vi "Convert_ERDs.vi"(0 "New Header?":bool, 2 "ERD Name":string[](array[string]), 5 "All_ERD_Data_Bundled_Brass In":T1, 7 "Array":T14[](array[typedef]) {"ERD Number" format="%.0x"}, 11 "Error In":errorcluster) -> (4 "All_ERD_Data_Bundled_Brass":T1, 15 "Error Out":errorcluster)   [LabVIEW 2021]
doc: "This VI parses the data from ERDs in correct format, units, etc. It handles all hex to dec conversions, hex to enum, and hex to boolean conversions.\n\nIf Raw Data from ERD is blank string, then it will output values from shift register."
uses:
  Common/LabVIEW GEA2 Toolkit/GEA3/type defs/ERD Read Data Out.ctl
  type defs/All_Bundled_Data.ctl
  type defs/Version.ctl
  type defs/ERD_Always_Show.ctl
  type defs/Brass Matrix.ctl
  type defs/CSV_File_String_Arrays.ctl
  type defs/Redundant.ctl
  type defs/Algorithms.ctl
  type defs/ATC_Data.ctl
  type defs/Fault Table Array.ctl
  type defs/Fault_Table_Info.ctl
  Dryer Tool (Commercial 2)/JL Dryer Tool Support/type defs/ERD_RJ45.ctl
  Dryer Tool (Commercial 2)/JL Dryer Tool Support/type defs/ERD_Commercial_Laundry.ctl
  type defs/BootloaderVersion.ctl
panel:
  out "x/y":dbl
  out "Data":string
  # "Wet Load Size"
  # "Dry Load Size"
  # "OOB"
  # "Wet Load Size"
  # "Dry Load Size"
  # "OOB"
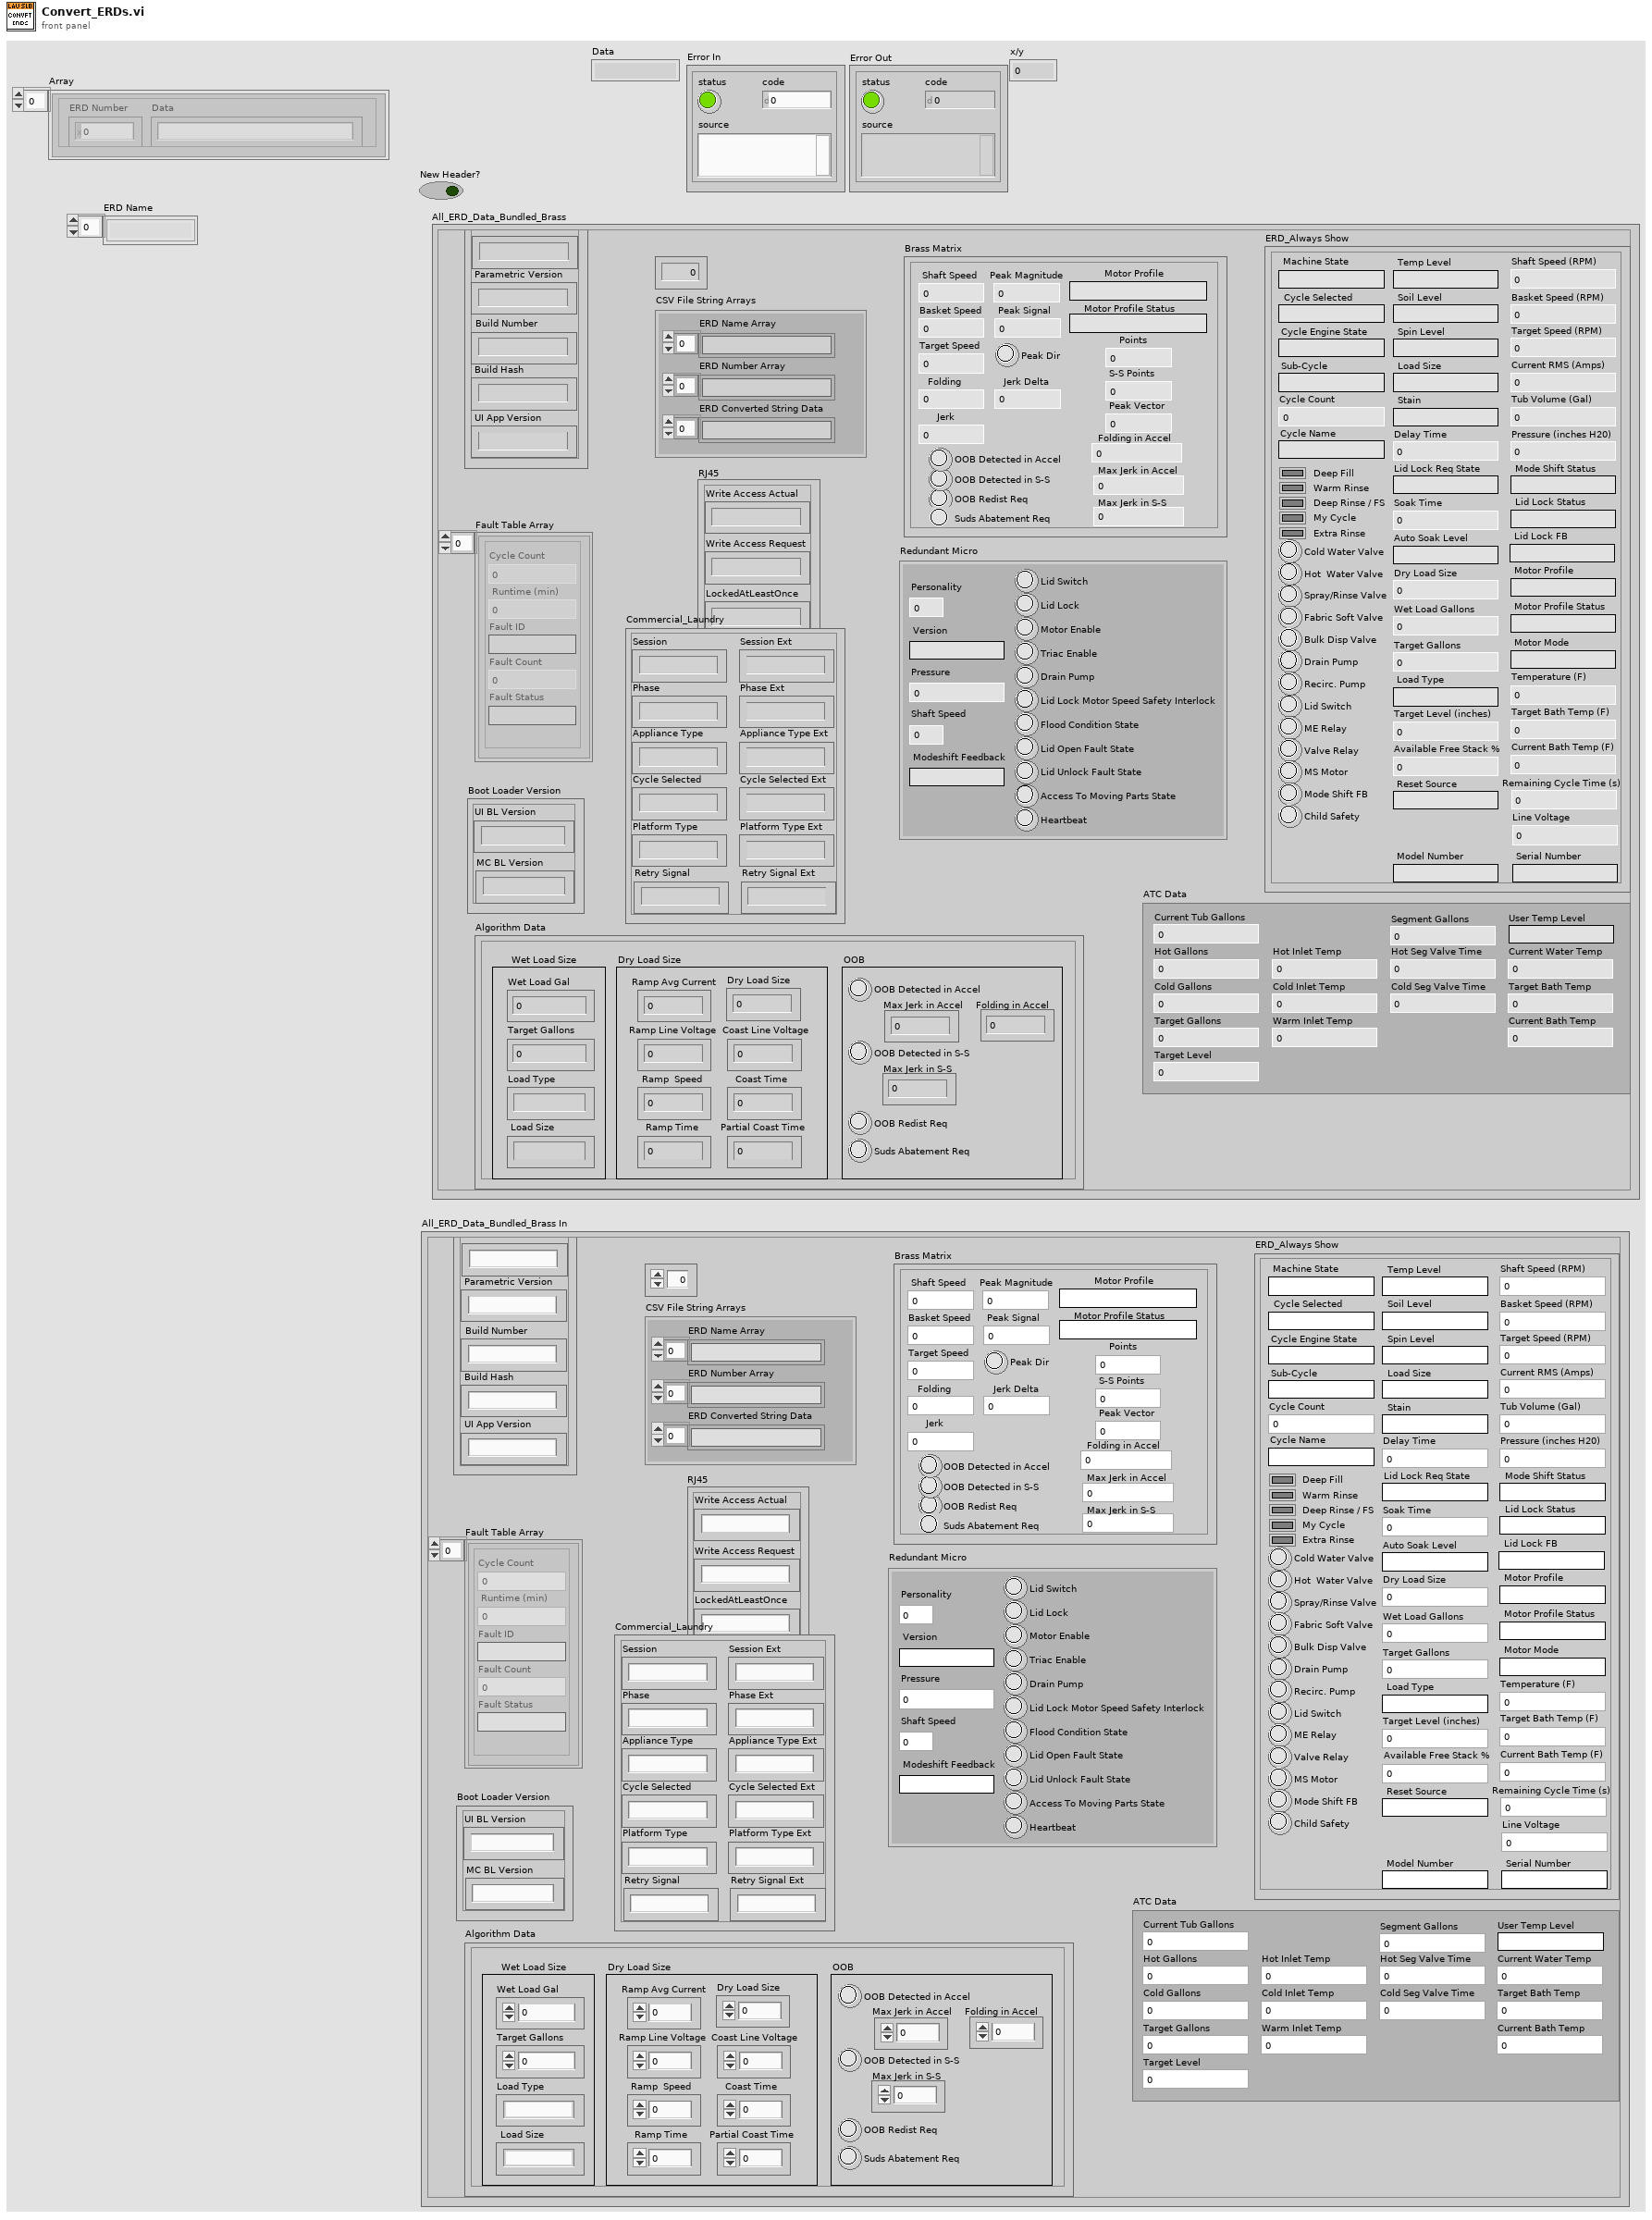
[diagram p1: front panel]
types:
  T1 = typedef "All_Bundled_Data.ctl" = cluster{"Software MC":T2, "ERD_Always Show":T3, "Personality Set":u8, "Brass Matrix":T4, "CSV File String Arrays":T5, "Redundant Micro":T6, "Algorithm Data":T7, "ATC Data":T8, "Fault Table Array ":T9, "RJ45":T11, "Commercial_Laundry":T12, "Boot Loader Version":T13}
  T2 = typedef "Version.ctl" = cluster{"Build Number":string, "Build Hash ":string, "Application Version":string, "Parametric Version":string, "UI App Version":string}
  T3 = typedef "ERD_Always_Show.ctl" = cluster{"Basket Speed (RPM)":u16, "Machine State":string, "Tub Volume (Gal)":dbl, "Pressure (inches H20)":dbl, "Lid Switch ":bool, "Current RMS (Amps)":dbl, "Cycle Selected":string, "Lid Lock Status":string, "Mode Shift Status":string, "Spray/Rinse Valve":bool, "Fabric Soft Valve":bool, "Drain Pump":bool, "Recirc. Pump":bool, "Cycle Engine State":string, "Hot  Water Valve":bool, "Cold Water Valve":bool, "Motor Profile":string, "Motor Profile Status":string, "Motor Mode":string, "ME Relay":bool, "Cycle Count":u32, "Deep Rinse / FS":bool, "My Cycle":bool, "Soil Level":string, "Spin Level":string, "Stain":string, "Temp Level":string, "Load Size":string, "Delay Time":u16, "Soak Time":u16, "Deep Fill":bool, "Warm Rinse":bool, "Auto Soak Level":string, "Extra Rinse":bool, "Wet Load Gallons":dbl, "Target Gallons":dbl, "Sub-Cycle":string, "Load Type":string, "Target Level (inches)":dbl, "Valve Relay":bool, "Dry Load Size":dbl, "Shaft Speed (RPM) ":u16, "MS Motor":bool, "Mode Shift FB":bool, "Target Bath Temp (F)":dbl, "Temperature (F)":dbl, "Current Bath Temp (F)":dbl, "Lid Lock FB":string, "Lid Lock Req State":string, "Remaining Cycle Time (s)":u32, "Available Free Stack %":u8, "Child Safety":bool, "Target Speed (RPM)":u16, "Reset Source":string, "Line Voltage":dbl, "Cycle Name":string, "Bulk Disp Valve":bool, "Model Number":string, "Serial Number":string}
  T4 = typedef "Brass Matrix.ctl" = cluster{"Shaft Speed":u16, "Folding":i32, "Jerk":i32, "Basket Speed":u16, "Target Speed":u16, "Peak Signal":u8, " Peak Magnitude":dbl, "Folding in Accel":i32, "Max Jerk in Accel":i32, "Max Jerk in S-S":i32, "Motor Profile Status":string, "Motor Profile":string, "OOB Redist Req":bool, "OOB Detected in S-S":bool, "OOB Detected in Accel":bool, "Suds Abatement Req ":bool, "Peak Dir":bool, "Peak Vector":dbl, "S-S Points":u8, "Points":u8, "Jerk Delta":i32}
  T5 = typedef "CSV_File_String_Arrays.ctl" = cluster{"ERD Number Array":string[], "ERD Name Array":string[], "ERD Converted String Data":string[]}
  T6 = typedef "Redundant.ctl" = cluster{"Version":string, "Personality":u8, "Pressure ":dbl, "Shaft Speed":u16, "Modeshift Feedback":string, "Lid Switch":bool, "Lid Lock":bool, "Triac Enable":bool, "Drain Pump":bool, "Lid Lock Motor Speed Safety Interlock":bool, "Flood Condition State":bool, "Lid Open Fault State":bool, "Access To Moving Parts State":bool, "Heartbeat":bool, "Motor Enable":bool, "Lid Unlock Fault State":bool}
  T7 = typedef "Algorithms.ctl" = cluster{"Wet Load Gal":dbl, "Target Gallons":dbl, "Load Type":string, "Load Size":string, "Coast Time":u16, "Ramp Time":u16, "Ramp  Speed":u16, "Ramp Avg Current":dbl, "OOB Redist Req":bool, "OOB Detected in S-S":bool, "Folding in Accel":i32, "Max Jerk in Accel":i32, "Max Jerk in S-S":i32, "OOB Detected in Accel":bool, "Partial Coast Time":u16, "Dry Load Size":dbl, "Ramp Line Voltage ":dbl, "Coast Line Voltage":dbl, "Suds Abatement Req ":bool}
  T8 = typedef "ATC_Data.ctl" = cluster{"Current Tub Gallons":dbl, "Hot Gallons":dbl, "Cold Gallons":dbl, "Target Gallons":dbl, "Current Water Temp":dbl, "Target Level":dbl, "Target Bath Temp":dbl, "Current Bath Temp ":dbl, "Cold Inlet Temp":dbl, "Hot Inlet Temp":dbl, "Warm Inlet Temp":dbl, "Hot Seg Valve Time":u16, "Cold Seg Valve Time ":u16, "User Temp Level":string, "Segment Gallons":dbl}
  T9 = typedef "Fault Table Array.ctl" = T10[]
  T10 = typedef "Fault_Table_Info.ctl" = cluster{"Cycle Count":u32, " Runtime (min) ":u32, "Fault Status":string, "Fault ID":string, "Fault Count":u16}
  T11 = typedef "ERD_RJ45.ctl" = cluster{"Write Access Actual":string, "Write Access Request":string, "LockedAtLeastOnce":string}
  T12 = typedef "ERD_Commercial_Laundry.ctl" = cluster{"Session":string, "Phase":string, "Appliance Type":string, "Cycle Selected":string, "Platform Type":string, "Retry Signal":string, "Session Ext":string, "Phase Ext":string, "Appliance Type Ext":string, "Cycle Selected Ext":string, "Platform Type Ext":string, "Retry Signal Ext":string}
  T13 = typedef "BootloaderVersion.ctl" = cluster{"UI BL Version":string, "MC BL Version":string}
  T14 = typedef "ERD Read Data Out.ctl" = cluster{"ERD Number":u16, "Data":string}
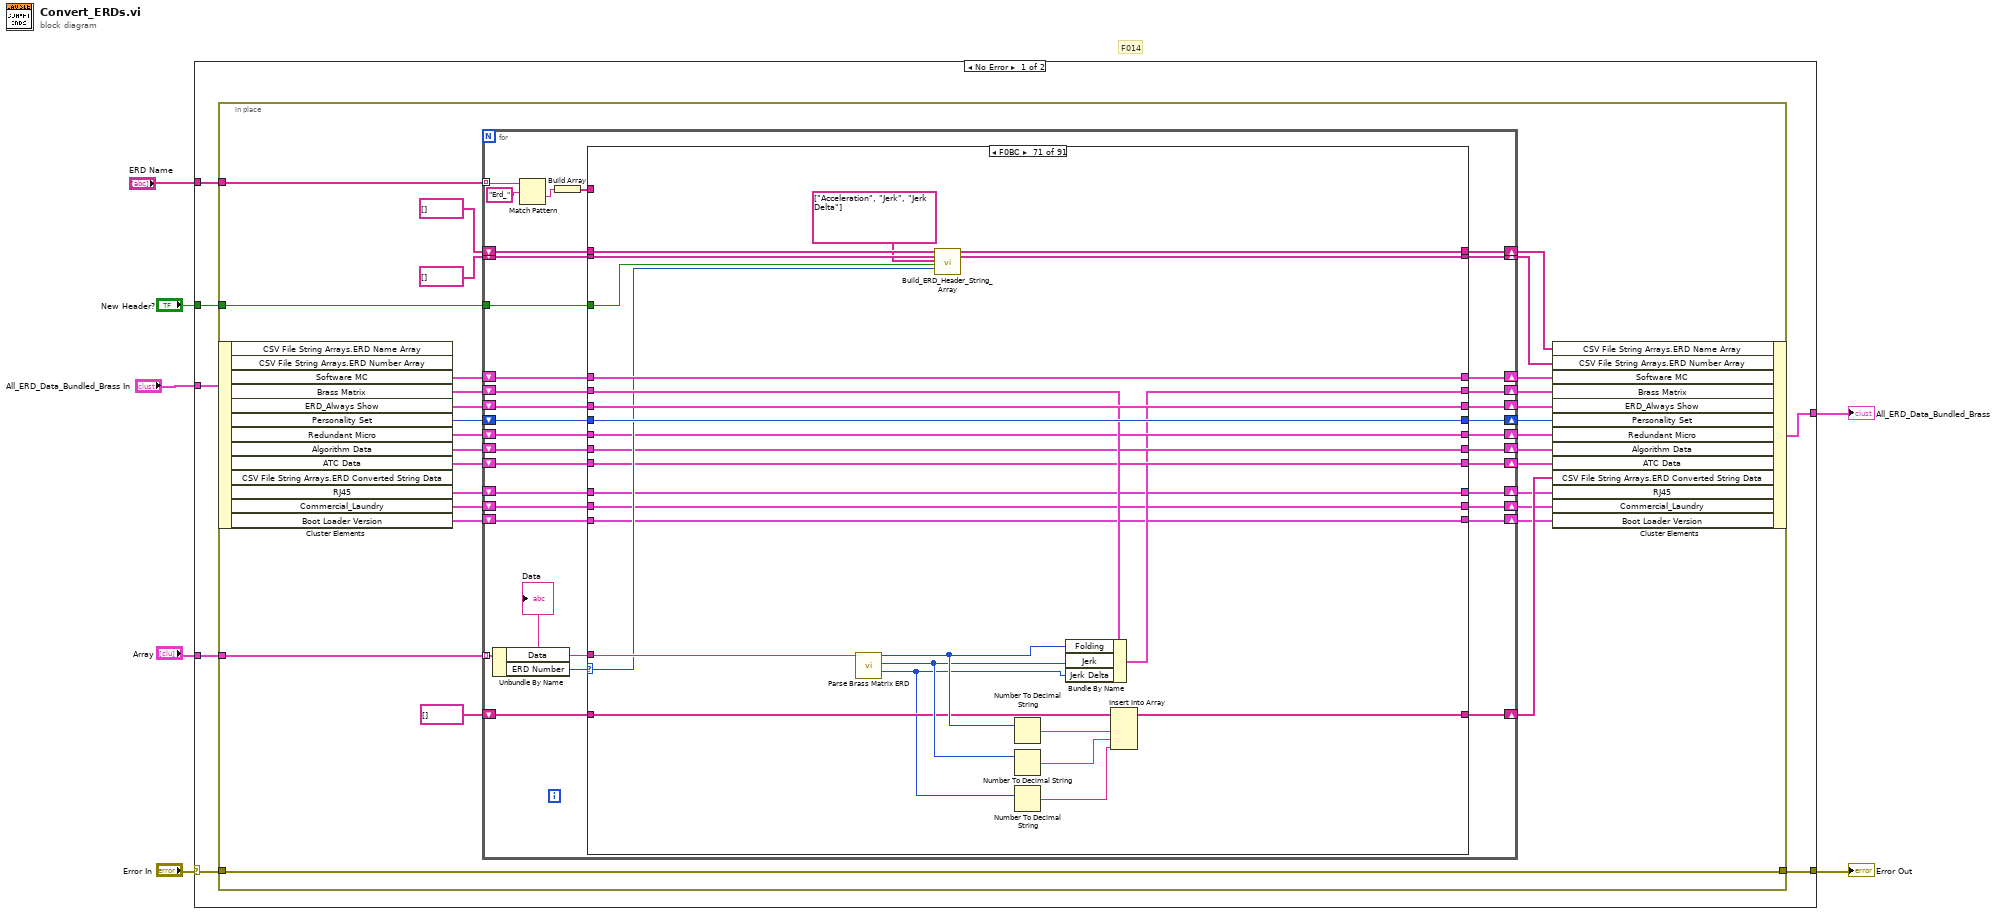
[diagram p0: block diagram]
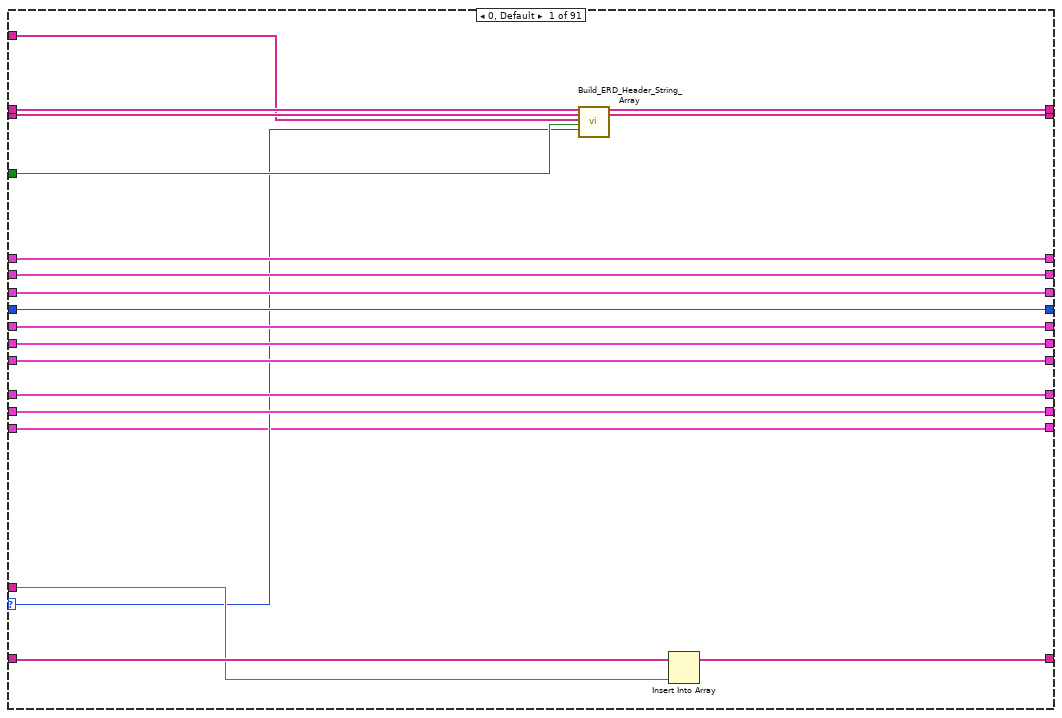
[diagram p2: hidden frame]
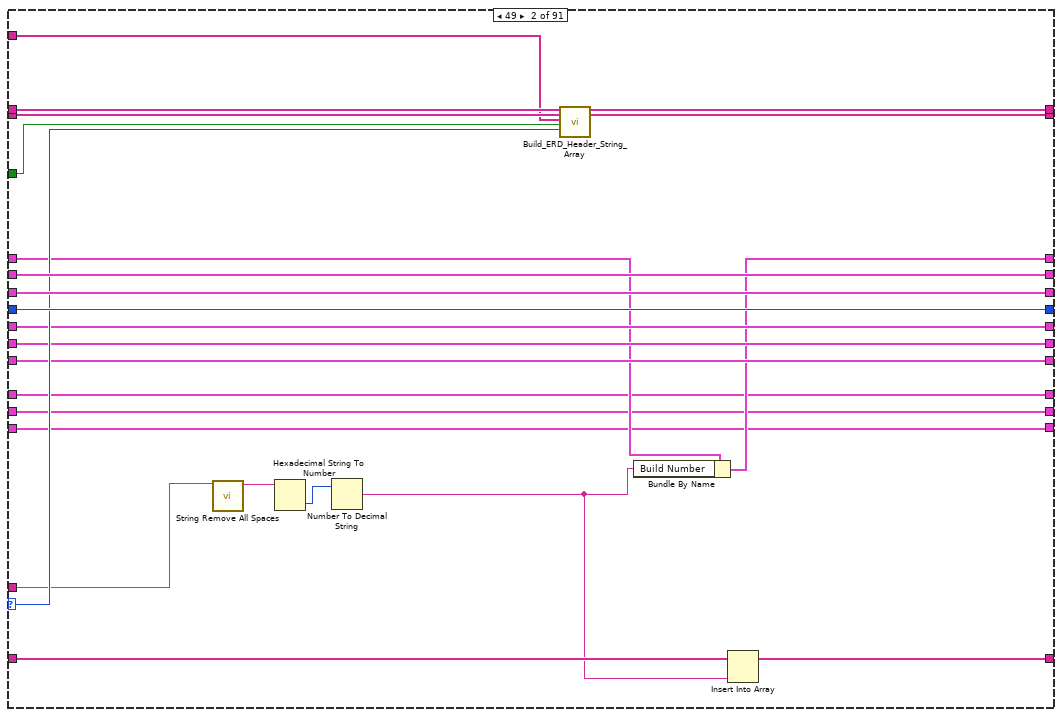
[diagram p3: hidden frame]
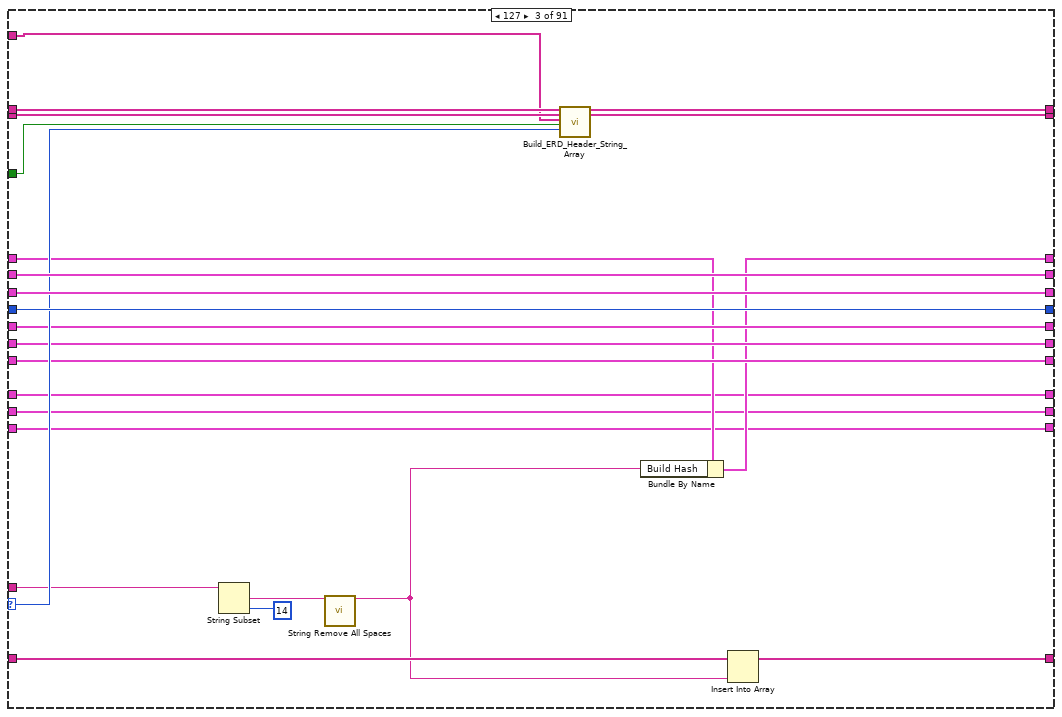
[diagram p4: hidden frame]
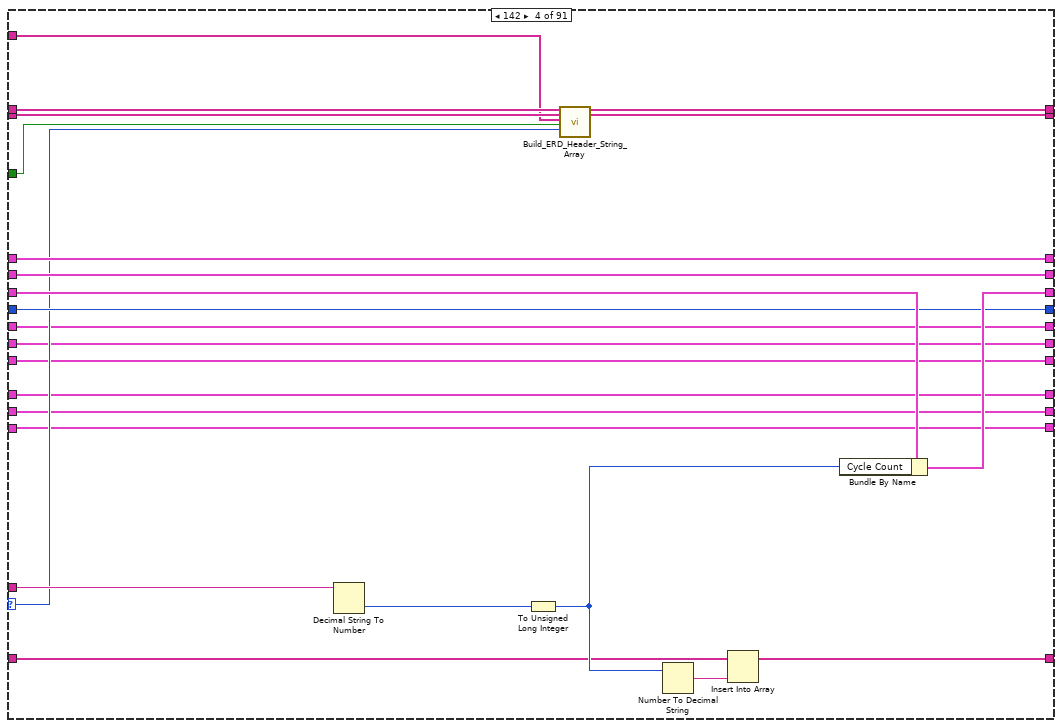
[diagram p5: hidden frame]
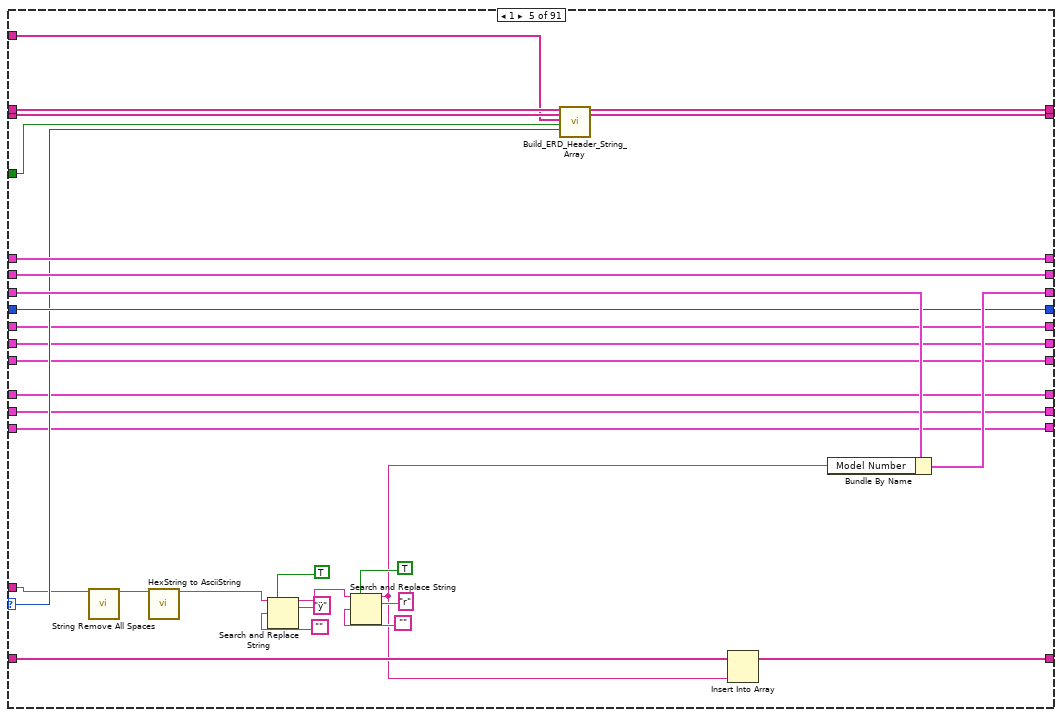
[diagram p6: hidden frame]
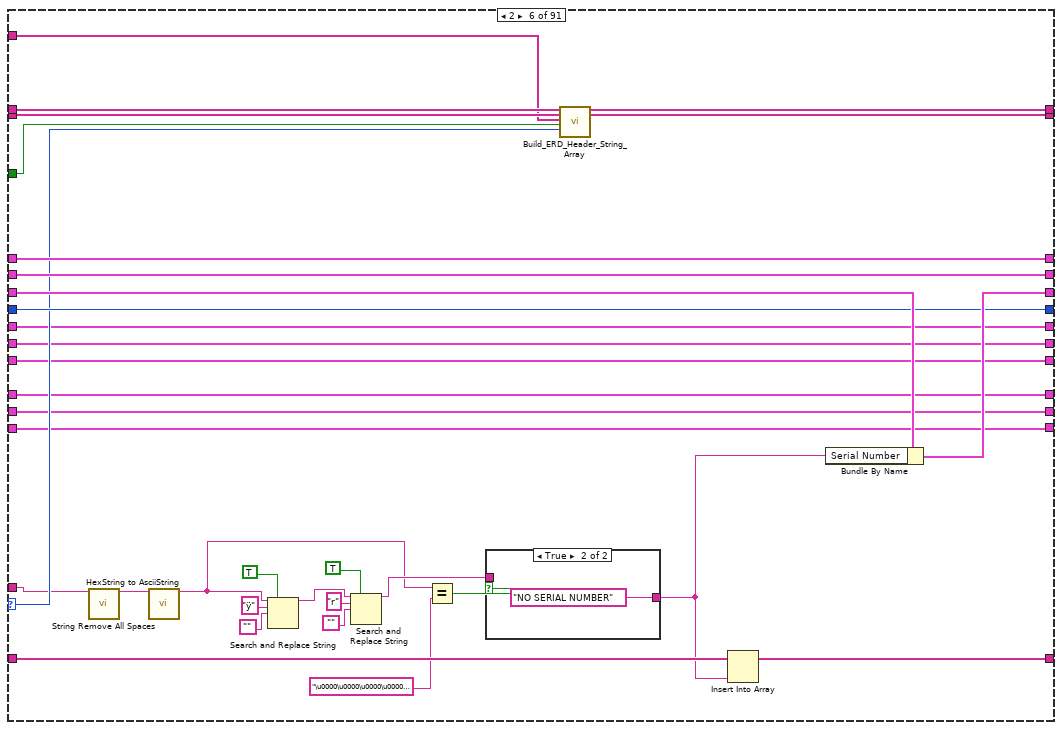
[diagram p7: hidden frame]
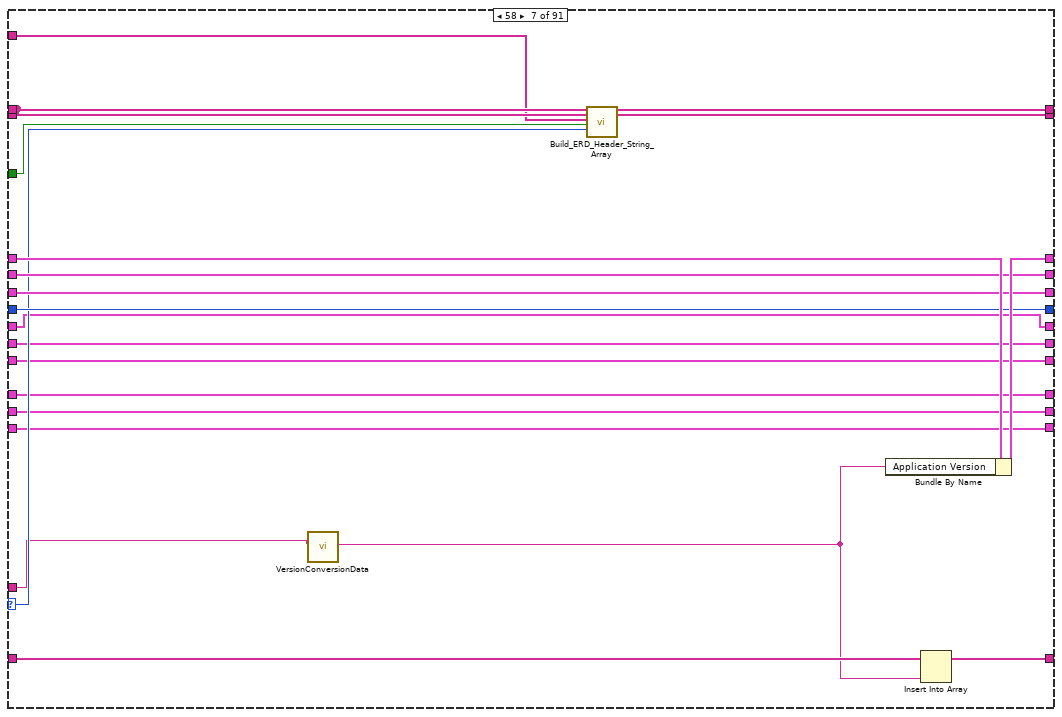
[diagram p9: hidden frame]
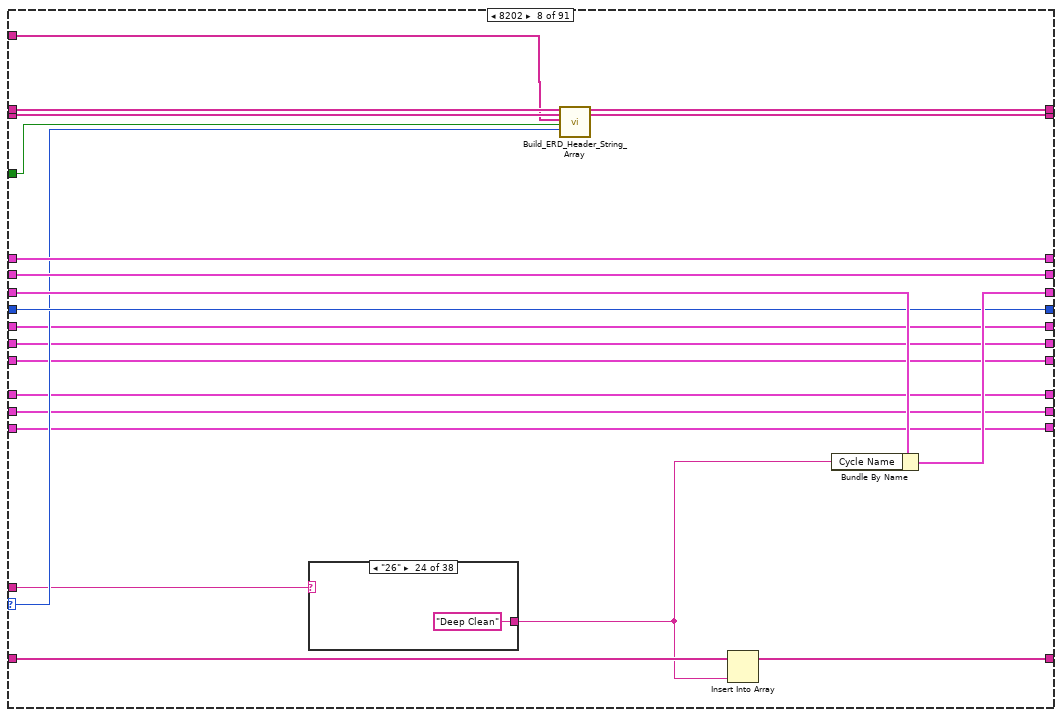
[diagram p10: hidden frame]
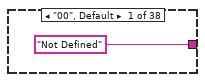
[diagram p11: hidden frame]
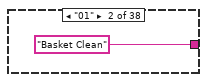
[diagram p12: hidden frame]
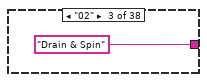
[diagram p13: hidden frame]
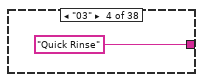
[diagram p14: hidden frame]
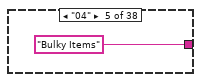
[diagram p15: hidden frame]
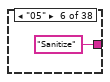
[diagram p16: hidden frame]
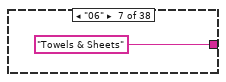
[diagram p17: hidden frame]
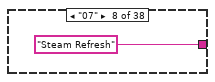
[diagram p18: hidden frame]
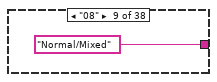
[diagram p19: hidden frame]
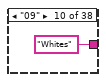
[diagram p20: hidden frame]
diagram:
  # "F014"
  n1 = case shown="No Error" "Error In" {
    selector: "Error In" -> [w11 w2792]
    tunnel: "Array" -> [w14 _]
    tunnel: [w12 w2791] -> w5
    tunnel: "All_ERD_Data_Bundled_Brass In" -> [w13 w2790]
    tunnel: [w10 w2790] -> w4
    tunnel: "New Header?" -> [w9 _]
    tunnel: "ERD Name" -> [w8 _]
    frame No Error {
      n2 = in-place {
        in-place-border: w14 -> [w44]
        in-place-border: [w40] -> w12
        in-place-border: w11 -> [w40]
        in-place-border: w9 -> [w33]
        in-place-border: w8 -> [w15]
        n3 = in-place-cluster #1(w13) -> ("Software MC"=w42:T2, "Brass Matrix"=w41:T4, "ERD_Always Show"=w43:T3, "Personality Set"=w36:u8, "Redundant Micro"=w26:T6, "Algorithm Data"=w25:T7, "ATC Data"=w23:T8, "RJ45"=w21:T11, "Commercial_Laundry"=w19:T12, "Boot Loader Version"=w17:T13)  [unwired: 3 out]
        n4 = for {
          tunnel: w44 -> [w78] mode=indexing
          shift-right: [w77] -> w37
          shift-left: w43 -> [w76]
          shift-right: [w74] -> w39
          shift-left: w42 -> [w75]
          shift-right: [w72] -> w38
          shift-left: w41 -> [w73]
          shift-right: [w69] -> w35
          shift-left: w36 -> [w70]
          shift-right: [w67] -> w28
          shift-left: string[] [] ("ERD String Data") -> [w68]
          tunnel: w33 -> [w66]
          shift-right: [w62] -> w29
          shift-left: string[] [] ("ERD String Data") -> [w65]
          shift-right: [w63] -> w30
          shift-left: string[] [] ("ERD String Data") -> [w64]
          shift-right: [w61] -> w27
          shift-left: w26 -> [w60]
          shift-right: [w58] -> w24
          shift-left: w25 -> [w59]
          shift-right: [w56] -> w22
          shift-left: w23 -> [w57]
          shift-right: [w54] -> w20
          shift-left: w21 -> [w55]
          shift-right: [w52] -> w18
          shift-left: w19 -> [w53]
          shift-right: [w50] -> w16
          shift-left: w17 -> [w51]
          tunnel: w15 -> [w47] mode=indexing
          n5 = Unbundle By Name(w78) -> ("Data"=w49:string, "ERD Number"=w71:u16)
          "Data" <- w49
          n6 = Match Pattern(string=w47, regular expression="Erd_") -> (after substring=w45:string)  [unwired: 1 in, 3 out]
          n7 = Build Array(w45) -> (w46:string[])
          n8 = case shown="F0BC" w71 {
            selector: w71 -> [w81 w114 w138 w159 w191 w225 w247 w270 w325 w349 w381 w401 w420 w444 w469 w494 w519 w550 w578 w610 w639 w672 w711 w733 w755 w783 w808 w841 w866 w900 w933 w955 w986 w1011 w1043 w1070 w1113 w1144 w1165 w1205 w1224 w1261 w1280 w1313 w1342 w1371 w1391 w1446 w1483 w1510 w1540 w1558 w1592 w1623 w1652 w1675 w1705 w1729 w1748 w1780 w1818 w1862 w1887 w1908 w1937 w1964 w2001 w2026 w2051 w2074 w2125 w2139 w2164 w2185 w2214 w2242 w2260 w2307 w2330 w2361 w2383 w2406 w2431 w2457 w2489 _ w2545 w2570 w2595 w2641 w2732]
            tunnel: w49 -> [w82 w102 w130 w170 w176 w206 w239 w264 w341 w362 w391 w392 w435 w458 w483 w508 w532 w560 w590 w622 w649 w685 w727 w741 w768 w800 w822 w827 w858 w892 w917 w969 w1004 w1030 w1058 w1084 w1104 w1156 w1182 w1192 w1242 w1246 w1300 w1304 w1333 w1382 w1411 w1459 w1495 w1502 w1552 w1575 w1604 w1614 w1644 w1691 w1715 w1739 w1767 w1790 w1828 w1847 w1875 w1922 w1950 w1980 w2015 w2040 w2065 w2088 w2128 w2152 w2179 w2204 w2229 w2252 w2277 w2286 w2344 w2368 w2379 w2402 w2440 w2453 w2502 w2512 w2536 w2561 w2586 w2609 w2700]
            tunnel: [w98 w122 w146 w168 w200 w234 w256 w279 w339 w363 w390 w411 w432 w459 w484 w509 w533 w561 w591 w621 w652 w687 w725 w748 w771 w798 w826 w854 w883 w913 w944 w967 w1003 w1025 w1056 w1095 w1131 w1154 w1181 w1217 w1240 w1273 w1298 w1332 w1361 w1387 w1433 w1475 w1494 w1528 w1550 w1576 w1607 w1641 w1670 w1694 w1718 w1743 w1765 w1807 w1845 w1873 w1897 w1925 w1947 w1982 w2013 w2038 w2063 w2097 w2131 w2153 w2177 w2202 w2227 w2255 w2282 w2319 w2342 w2373 w2398 w2421 w2444 w2467 w2504 w2513 w2554 w2579 w2604 w2650 w2741] -> w77
            tunnel: w76 -> [w98 w122 w146 w169 w201 w235 w256 w280 w340 w364 w390 w411 w434 w460 w485 w510 w534 w562 w592 w623 w651 w686 w726 w749 w772 w799 w821 w855 w884 w914 w945 w968 w1005 w1026 w1057 w1096 w1132 w1155 w1183 w1218 w1241 w1274 w1299 w1332 w1361 w1387 w1433 w1475 w1496 w1528 w1551 w1577 w1608 w1641 w1670 w1694 w1718 w1743 w1766 w1807 w1845 w1874 w1899 w1926 w1948 w1983 w2013 w2038 w2063 w2096 w2131 w2154 w2178 w2203 w2228 w2255 w2282 w2319 w2342 w2373 w2398 w2421 w2444 w2468 w2505 w2513 w2554 w2579 w2604 w2650 w2741]
            tunnel: w75 -> [w97 w108 w132 w167 w199 w233 w258 w278 w338 w361 w389 w413 w437 w457 w482 w507 w531 w559 w589 w620 w648 w684 w724 w747 w770 w797 w825 w853 w882 w912 w943 w966 w1002 w1027 w1055 w1082 w1130 w1153 w1180 w1216 w1239 w1272 w1297 w1331 w1360 w1386 w1432 w1474 w1498 w1527 w1549 w1574 w1603 w1640 w1669 w1693 w1717 w1742 w1764 w1808 w1846 w1872 w1898 w1920 w1949 w1979 w2014 w2039 w2064 w2087 w2130 w2151 w2176 w2201 w2226 w2254 w2281 w2318 w2343 w2372 w2397 w2420 w2443 w2482 w2501 w2516 w2541 w2566 w2591 w2638 w2729]
            tunnel: [w97 w107 w131 w167 w199 w233 w257 w278 w338 w361 w389 w412 w437 w457 w482 w507 w531 w559 w589 w620 w648 w684 w724 w747 w770 w797 w825 w853 w882 w912 w943 w966 w1002 w1027 w1055 w1082 w1130 w1153 w1180 w1216 w1239 w1272 w1297 w1331 w1360 w1386 w1432 w1474 w1498 w1527 w1549 w1574 w1603 w1640 w1669 w1693 w1717 w1742 w1764 w1808 w1846 w1872 w1898 w1920 w1949 w1979 w2014 w2039 w2064 w2087 w2130 w2151 w2176 w2201 w2226 w2254 w2281 w2318 w2343 w2372 w2397 w2420 w2443 w2482 w2501 w2516 w2541 w2566 w2591 w2638 w2729] -> w74
            tunnel: w73 -> [w96 w121 w145 w166 w198 w232 w255 w277 w337 w360 w388 w410 w436 w456 w481 w506 w530 w558 w588 w619 w647 w683 w723 w746 w769 w796 w824 w840 w881 w911 w942 w965 w1001 w1028 w1054 w1081 w1129 w1152 w1179 w1215 w1238 w1271 w1296 w1329 w1358 w1381 w1410 w1456 w1497 w1526 w1548 w1573 w1602 w1642 w1671 w1695 w1719 w1741 w1763 w1806 w1844 w1870 w1895 w1919 w1945 w1978 w2012 w2037 w2062 w2085 w2127 w2150 w2175 w2200 w2213 w2256 w2268 w2306 w2341 w2370 w2382 w2405 w2442 w2481 w2500 w2532 w2553 w2578 w2603 w2649 w2740]
            tunnel: [w96 w121 w145 w166 w198 w232 w255 w277 w337 w360 w388 w410 w436 w456 w481 w506 w530 w558 w588 w619 w647 w683 w723 w746 w769 w796 w824 w840 w881 w911 w942 w965 w1001 w1028 w1054 w1081 w1129 w1152 w1179 w1215 w1238 w1271 w1296 w1329 w1358 w1381 w1410 w1456 w1497 w1526 w1548 w1573 w1602 w1642 w1671 w1695 w1719 w1741 w1763 w1805 w1843 w1869 w1894 w1919 w1944 w1978 w2011 w2036 w2061 w2084 w2110 w2150 w2175 w2200 w2213 w2256 w2268 w2305 w2340 w2369 w2381 w2404 w2442 w2481 w2500 w2532 w2553 w2578 w2603 w2649 w2740] -> w72
            tunnel: w70 -> [w95 w120 w144 w165 w197 w231 w254 w276 w336 w359 w387 w409 w431 w455 w480 w505 w529 w557 w587 w618 w646 w682 w722 w745 w767 w795 w820 w852 w880 w910 w941 w964 w1000 w1024 w1053 w1080 w1128 w1151 w1178 w1214 w1237 w1270 w1295 w1328 w1357 w1380 w1409 w1455 w1493 w1525 w1547 w1572 w1599 w1638 w1667 w1690 w1714 w1738 w1762 w1789 w1827 w1871 w1896 w1918 w1946 w1977 w2010 w2035 w2060 w2086 w2129 w2149 w2174 w2199 w2225 w2251 w2276 w2317 w2339 w2371 w2395 w2418 _ w2480 w2499 w2531 w2552 w2577 w2602 w2648 w2739]
            tunnel: [w95 w120 w144 w165 w197 w231 w254 w276 w336 w359 w387 w409 w431 w455 w480 w505 w529 w557 w587 w618 w646 w682 w722 w745 w767 w795 w820 w852 w880 w910 w941 w964 w1000 w1024 w1053 w1080 w1128 w1151 w1178 w1214 w1237 w1270 w1295 w1328 w1357 w1380 w1409 w1455 w1493 w1525 w1547 w1572 w1599 w1638 w1667 w1690 w1714 w1738 w1762 w1789 w1827 w1871 w1896 w1918 w1946 w1977 w2010 w2035 w2060 w2086 w2129 w2149 w2174 w2199 w2225 w2251 w2276 w2317 w2339 w2371 w2395 w2418 w2427 w2480 w2499 w2531 w2552 w2577 w2602 w2648 w2739] -> w69
            tunnel: w68 -> [w87 w118 w142 w163 w195 w229 _ w274 w329 w353 w385 w405 w427 w448 w473 w498 w523 w554 w584 w614 w643 w676 w715 w739 w759 w787 w812 w845 w870 w904 w937 w959 w990 w1018 w1047 w1074 w1117 w1148 w1169 w1209 w1228 w1265 w1288 w1323 w1346 w1375 w1401 w1450 w1487 w1520 w1544 w1566 w1596 w1627 w1656 w1679 w1709 w1733 w1752 w1784 w1822 w1866 w1891 w1912 w1941 w1968 w2005 w2030 w2055 w2078 w2126 w2143 w2168 w2189 w2218 w2246 w2271 w2312 w2334 w2365 w2387 w2410 w2435 w2461 w2493 w2526 w2547 w2572 w2597 w2643 w2734]
            tunnel: [w85 w116 w140 w161 w193 w227 w249 w272 w327 w351 w383 w403 w425 w446 w471 w496 w521 w552 w582 w612 w641 w674 w713 w737 w757 w785 w810 w843 w868 w902 w935 w957 w988 w1016 w1045 w1072 w1115 w1146 w1167 w1207 w1226 w1263 w1286 w1321 w1344 w1373 w1399 w1448 w1485 w1518 w1542 w1564 w1594 w1625 w1654 w1677 w1707 w1731 w1750 w1782 w1820 w1864 w1889 w1910 w1939 w1966 w2003 w2028 w2053 w2076 w2123 w2141 w2166 w2187 w2216 w2244 w2269 w2310 w2332 w2363 w2385 w2408 w2433 w2459 w2491 w2523 w2543 w2568 w2593 w2639 w2730] -> w67
            tunnel: w66 -> [w89 w115 w139 w160 w192 w226 w248 w271 w326 w350 w382 w402 w424 w445 w470 w495 w520 w551 w579 w611 w640 w673 w712 w734 w756 w784 w809 w842 w867 w901 w934 w956 w987 w1012 w1044 w1071 w1114 w1145 w1166 w1206 w1225 w1262 w1281 w1314 w1343 w1372 w1392 w1447 w1484 w1511 w1541 w1559 w1593 w1624 w1653 w1676 w1706 w1730 w1749 w1781 w1819 w1863 w1888 w1909 w1938 w1965 w2002 w2027 w2052 w2075 w2124 w2140 w2165 w2186 w2215 w2243 w2261 w2309 w2331 w2362 w2384 w2407 w2432 w2458 w2490 w2525 w2546 w2571 w2596 w2642 w2733]
            tunnel: w65 -> [w88 w119 w143 w164 w196 w230 w251 w275 w330 w354 w386 w406 w428 w449 w474 w499 w524 w555 w585 w615 w644 w677 w716 w740 w760 w788 w813 w846 w871 w905 w938 w961 w991 w1019 w1048 w1075 w1118 w1149 w1170 w1210 w1229 w1266 w1289 w1324 w1347 w1376 w1402 w1451 w1488 w1521 w1545 w1567 w1597 w1628 w1657 w1680 w1710 w1734 w1753 w1785 w1823 w1867 w1892 w1913 w1942 w1969 w2006 w2031 w2056 w2079 w2122 w2144 w2169 w2190 w2219 w2247 w2272 w2313 w2335 w2366 w2388 w2411 w2436 w2462 w2494 w2527 w2548 w2573 w2598 w2644 w2735]
            tunnel: w64 -> [w83 w113 w137 w155 w190 w224 w253 w269 w333 w357 w380 w408 w430 w452 w477 w502 w527 w549 w581 w609 w638 w680 w719 w743 w764 w792 w817 w849 w875 w898 w927 w951 w995 w1015 w1042 w1069 w1122 w1139 w1174 w1201 w1233 w1258 w1284 w1317 w1353 w1367 w1394 w1441 w1481 w1514 w1538 w1562 w1591 w1632 w1661 w1684 w1701 w1725 w1756 w1776 w1816 w1858 w1882 w1906 w1932 w1973 w1998 w2023 w2048 w2073 w2114 w2137 w2161 w2194 w2222 w2238 w2264 w2303 w2327 w2355 w2391 w2414 w2429 w2456 w2488 w2522 w2538 w2563 w2588 w2637 w2728]
            tunnel: [w84 w112 w136 w154 w189 w223 w252 w268 w332 w356 w379 w407 w423 w451 w476 w501 w526 w548 w580 w608 w637 w679 w718 w742 w763 w791 w816 w848 w874 w897 w926 w952 w994 w1014 w1041 w1068 w1121 w1138 w1173 w1200 w1232 w1257 w1283 w1316 w1352 w1366 w1393 w1440 w1480 w1513 w1537 w1561 w1590 w1631 w1660 w1683 w1700 w1724 w1755 w1775 w1815 w1857 w1881 w1905 w1930 w1972 w1997 w2022 w2047 w2071 w2113 w2136 w2160 w2193 w2221 w2237 w2263 w2302 w2326 w2354 w2390 w2413 w2428 w2455 w2487 w2521 w2537 w2562 w2587 w2636 w2727] -> w63
            tunnel: [w86 w117 w141 w162 w194 w228 w250 w273 w328 w352 w384 w404 w426 w447 w472 w497 w522 w553 w583 w613 w642 w675 w714 w738 w758 w786 w811 w844 w869 w903 w936 w958 w989 w1017 w1046 w1073 w1116 w1147 w1168 w1208 w1227 w1264 w1287 w1322 w1345 w1374 w1400 w1449 w1486 w1519 w1543 w1565 w1595 w1626 w1655 w1678 w1708 w1732 w1751 w1783 w1821 w1865 w1890 w1911 w1940 w1967 w2004 w2029 w2054 w2077 w2119 w2142 w2167 w2188 w2217 w2245 w2270 w2311 w2333 w2364 w2386 w2409 w2434 w2460 w2492 w2524 w2544 w2569 w2594 w2640 w2731] -> w62
            tunnel: [w94 w111 w135 w153 w188 w222 w246 w267 w335 w358 w378 w400 w429 w454 w479 w504 w528 w556 w586 w617 w645 w681 w721 w744 w766 w794 w819 w851 w879 w909 w940 w963 w999 w1023 w1052 w1079 w1127 w1142 w1177 w1213 w1236 w1269 w1294 w1327 w1356 w1379 w1408 w1454 w1492 w1524 w1535 w1571 w1586 w1637 w1666 w1689 w1713 w1737 w1761 w1788 w1826 w1861 w1885 w1917 w1935 w1976 w2009 w2034 w2059 w2083 w2117 w2148 w2173 w2198 w2224 w2250 w2275 w2316 w2338 w2358 w2394 w2417 w2439 w2466 w2498 w2530 w2551 w2576 w2601 w2647 w2738] -> w61
            tunnel: w60 -> [w94 w111 w135 w153 w188 w222 w246 w267 w335 w358 _ w400 w429 w454 w479 w504 w528 w556 w586 w617 w645 w681 w721 w744 w766 w794 w819 w851 w879 w909 w940 w963 w999 w1023 w1052 w1079 w1127 w1142 w1177 w1213 w1236 w1269 w1294 w1327 w1356 w1379 w1408 w1454 w1492 w1524 w1535 w1571 w1586 w1637 w1666 w1689 w1713 w1737 w1761 w1788 w1826 w1861 w1885 w1917 w1935 w1976 w2009 w2034 w2059 w2083 w2117 w2148 w2173 w2198 w2224 w2250 w2275 w2316 w2338 w2358 w2394 w2417 w2439 w2466 w2498 w2530 w2551 w2576 w2601 w2647 w2738]
            tunnel: w59 -> [w93 w110 w134 w152 w187 w221 w245 w266 w324 w348 w377 w399 w419 w443 w468 w493 w518 w546 w577 w606 w635 w671 w710 w736 w754 w782 w807 w839 w878 w908 w930 w954 w998 w1022 w1051 w1078 w1126 w1141 w1176 w1212 w1235 w1268 w1293 w1326 w1355 w1378 w1407 w1453 w1491 w1523 w1534 w1570 w1585 w1635 w1664 w1687 w1704 w1728 w1759 w1779 w1814 w1860 w1884 w1916 w1934 w1975 w1996 w2021 w2046 w2082 w2116 w2147 w2172 w2197 w2212 w2241 w2267 w2315 w2325 w2357 w2392 w2415 w2438 w2465 w2497 w2529 w2550 w2575 w2600 w2646 w2737]
            tunnel: [w93 w110 w134 w152 w187 w221 w245 w266 w324 w348 w377 w399 w419 w443 w468 w493 w518 w546 w577 w605 w635 w671 w710 w736 w754 w782 w807 w838 w878 w908 w929 w953 w998 w1022 w1051 w1078 w1126 w1141 w1176 w1212 w1235 w1268 w1293 w1326 w1355 w1378 w1407 w1453 w1491 w1523 w1534 w1570 w1585 w1634 w1663 w1686 w1703 w1727 w1758 w1778 w1813 w1860 w1884 w1916 w1934 w1975 w1995 w2020 w2045 w2082 w2116 w2147 w2172 w2197 w2212 w2240 w2266 w2315 w2324 w2357 w2392 w2415 w2438 w2465 w2497 w2529 w2550 w2575 w2600 w2646 w2737] -> w58
            tunnel: w57 -> [w92 w109 w133 w151 w186 w220 w244 w265 w323 w347 w376 w398 w418 w442 w467 w492 w517 w545 w576 w607 w634 w670 w709 w735 w753 w781 w806 w836 w877 w907 w932 w962 w997 w1021 w1050 w1077 w1125 w1140 w1175 w1204 w1234 w1260 w1292 w1320 w1351 w1370 w1405 w1444 w1490 w1517 w1533 w1569 w1584 w1636 w1665 w1688 w1712 w1736 w1760 w1787 w1825 w1859 w1883 w1915 w1933 w1974 w2008 w2033 w2058 w2081 w2115 w2146 w2171 w2196 w2210 w2249 w2274 w2314 w2337 w2356 w2393 w2416 w2437 w2464 w2496 w2528 w2549 w2574 w2599 w2645 w2736]
            tunnel: [w92 w109 w133 w151 w186 w220 w244 w265 w323 w347 w376 w398 w418 w442 w467 w492 w517 w545 w575 w607 w634 w670 w709 w735 w753 w781 w806 w836 w877 w907 w931 w962 w997 w1021 w1050 w1077 w1124 w1140 w1175 w1203 w1234 w1259 w1291 w1319 w1350 w1369 w1406 w1445 w1490 w1516 w1533 w1569 w1584 w1636 w1665 w1688 w1712 w1736 w1760 w1787 w1825 w1859 w1883 w1915 w1933 w1974 w2008 w2033 w2058 w2081 w2115 w2146 w2171 w2196 w2210 w2249 w2274 w2314 w2337 w2356 w2393 w2416 w2437 w2464 w2496 w2528 w2549 w2574 w2599 w2645 w2736] -> w56
            tunnel: w55 -> [w91 w106 w126 w150 w174 w211 w243 w262 w322 w346 w375 w397 w417 w441 w466 w491 w516 w544 w573 w603 w633 w669 w708 w732 w752 w780 w805 w835 w865 w895 w924 w949 w985 w1010 w1039 w1065 w1112 w1136 w1164 w1199 w1223 w1254 w1279 w1312 w1341 w1364 w1390 w1436 w1478 w1509 w1532 w1557 w1582 w1622 w1651 w1674 w1698 w1722 w1746 w1773 w1811 w1855 w1879 w1903 w1929 w1963 w1993 w2018 w2043 w2068 w2107 w2134 w2159 w2184 w2209 w2235 w2259 w2287 w2322 w2347 w2378 w2401 w2426 w2447 w2485 w2520 w2540 w2565 w2590 w2632 w2723]
            tunnel: [w91 w106 w126 w150 w174 w211 w243 w262 w322 w346 w375 w397 w417 w441 w466 w491 w516 w544 w573 w603 w633 w669 w708 w732 w752 w780 w805 w835 w865 w895 w924 w949 w985 w1010 w1039 w1065 w1112 w1136 w1164 w1199 w1223 w1254 w1279 w1312 w1341 w1364 w1390 w1436 w1478 w1509 w1532 w1557 w1582 w1622 w1651 w1674 w1698 w1722 w1746 w1773 w1811 w1855 w1879 w1903 w1929 w1963 w1993 w2018 w2043 w2068 w2107 w2134 w2159 w2184 w2209 w2235 w2259 w2287 w2322 w2347 w2378 w2401 w2426 w2447 w2485 w2520 w2539 w2564 w2589 w2632 w2723] -> w54
            tunnel: w53 -> [w90 w105 w125 w149 w173 w210 w242 w261 w321 w345 w374 w396 w416 w440 w465 w490 w515 w543 w572 w602 w632 w668 w707 w731 w751 w779 w804 w834 w864 w894 w923 w948 w984 w1009 w1038 w1064 w1111 w1135 w1163 w1198 w1222 w1253 w1278 w1311 w1340 w1363 w1389 w1435 w1477 w1508 w1531 w1556 w1581 w1621 w1650 w1673 w1697 w1721 w1745 w1772 w1810 w1854 w1878 w1902 w1928 w1962 w1992 w2017 w2042 w2067 w2106 w2133 w2158 w2183 w2208 w2234 w2258 w2284 w2321 w2346 w2377 w2400 w2425 w2446 w2484 w2519 w2542 w2567 w2592 w2631 w2722]
            tunnel: [w90 w105 w125 w149 w173 w210 w242 w261 w321 w345 w374 w396 w416 w440 w465 w490 w515 w543 w572 w602 w632 w668 w707 w731 w751 w779 w804 w834 w864 w894 w923 w948 w984 w1009 w1038 w1064 w1111 w1135 w1163 w1198 w1222 w1253 w1278 w1311 w1340 w1363 w1389 w1435 w1477 w1508 w1531 w1556 w1581 w1621 w1650 w1673 w1697 w1721 w1745 w1772 w1810 w1854 w1878 w1902 w1928 w1962 w1992 w2017 w2042 w2067 w2106 w2133 w2158 w2183 w2208 w2234 w2258 w2284 w2321 w2346 w2377 w2400 w2425 w2446 w2484 w2519 w2542 w2567 w2592 w2630 w2721] -> w52
            tunnel: w51 -> [w80 w104 w124 w148 w172 w203 w241 w260 w320 w344 w373 w395 w415 w439 w464 w489 w514 w542 w571 w601 w631 w667 w706 w730 w750 w778 w803 w833 w863 w893 w922 w947 w983 w1008 w1037 w1063 w1110 w1134 w1162 w1197 w1221 w1252 w1277 w1310 w1339 w1362 w1388 w1434 w1476 w1507 w1530 w1555 w1580 w1620 w1649 w1672 w1696 w1720 w1744 w1771 w1809 w1853 w1877 w1901 w1927 w1961 w1991 w2016 w2041 w2066 w2105 w2132 w2157 w2182 w2207 w2233 w2257 w2283 w2320 w2345 w2376 w2399 w2422 w2445 w2483 w2515 w2535 w2560 w2585 w2635 w2726]
            tunnel: [w80 w104 w124 w148 w172 w203 w241 w260 w320 w344 w373 w395 w415 w439 w464 w489 w514 w542 w571 w601 w631 w667 w706 w730 w750 w778 w803 w833 w863 w893 w922 w947 w983 w1008 w1037 w1063 w1110 w1134 w1162 w1197 w1221 w1252 w1277 w1310 w1339 w1362 w1388 w1434 w1476 w1507 w1530 w1555 w1580 w1620 w1649 w1672 w1696 w1720 w1744 w1771 w1809 w1853 w1877 w1901 w1927 w1961 w1991 w2016 w2041 w2066 w2105 w2132 w2157 w2182 w2207 w2233 w2257 w2283 w2320 w2345 w2376 w2399 w2422 w2445 w2483 w2514 w2535 w2560 w2585 w2635 w2726] -> w50
            tunnel: w46 -> [w79 w103 w123 w147 w171 w202 w240 w259 w319 w343 w372 w394 w414 w438 w463 w488 w513 w541 w570 _ w630 w666 w705 w729 _ _ _ _ _ _ _ _ _ _ _ _ _ _ _ _ _ _ _ _ _ _ _ _ _ _ _ _ _ _ _ _ _ _ _ _ _ _ _ _ _ _ _ _ _ _ _ _ _ _ _ _ _ _ _ _ _ _ _ _ _ _ w2534 w2559 w2584 w2608 w2699]
            frame 0, Default {
              n9 = call "Build_ERD_Header_String_Array.vi"("ERD Name Array In"=w88, "ERD Number Array In"=w87, "ERD Name List"=w79, "New Header?"=w89, "ERD Number"=w81) -> ("ERD Name Array Out"=w86:string[], "ERD Number Array Out"=w85:string[])  [unwired: 13 in]
              n10 = Insert Into Array(array=w83, new element=w82) -> (w84:string[])  [unwired: 1 in]
            }
            frame 49 {
              n11 = call "String Remove All Spaces.vi"("Input String"=w102) -> ("Spaces Removed"=w101:string)  [unwired: 13 in, 1 out]
              n12 = Hexadecimal String To Number(string=w101) -> (number=w100:u32)  [unwired: 2 in, 1 out]
              n13 = Number To Decimal String(number=w100) -> (decimal integer string=w99:string)  [unwired: 1 in]
              n14 = call "Build_ERD_Header_String_Array.vi"("ERD Name Array In"=w119, "ERD Number Array In"=w118, "ERD Name List"=w103, "New Header?"=w115, "ERD Number"=w114) -> ("ERD Name Array Out"=w117:string[], "ERD Number Array Out"=w116:string[])  [unwired: 13 in]
              n15 = Bundle By Name(cluster=w108, "Build Number"=w99) -> (w107:T2)
              n16 = Insert Into Array(array=w113, new element=w99) -> (w112:string[])  [unwired: 1 in]
            }
            frame 127 {
              n17 = String Subset(string=w130, length (rest)=14 ("length (rest)")) -> (substring=w128:string)  [unwired: 1 in]
              n18 = call "String Remove All Spaces.vi"("Input String"=w128) -> ("Spaces Removed"=w127:string)  [unwired: 13 in, 1 out]
              n19 = call "Build_ERD_Header_String_Array.vi"("ERD Name Array In"=w143, "ERD Number Array In"=w142, "ERD Name List"=w123, "New Header?"=w139, "ERD Number"=w138) -> ("ERD Name Array Out"=w141:string[], "ERD Number Array Out"=w140:string[])  [unwired: 13 in]
              n20 = Bundle By Name(cluster=w132, "Build Hash"=w127) -> (w131:T2)
              n21 = Insert Into Array(array=w137, new element=w127) -> (w136:string[])  [unwired: 1 in]
            }
            frame 142 {
              n22 = Decimal String To Number(string=w170) -> (number=w157:i32)  [unwired: 2 in, 1 out]
              n23 = To Unsigned Long Integer(number=w157) -> (unsigned 32bit integer=w156:u32)
              n24 = call "Build_ERD_Header_String_Array.vi"("ERD Name Array In"=w164, "ERD Number Array In"=w163, "ERD Name List"=w147, "New Header?"=w160, "ERD Number"=w159) -> ("ERD Name Array Out"=w162:string[], "ERD Number Array Out"=w161:string[])  [unwired: 13 in]
              n25 = Number To Decimal String(number=w156) -> (decimal integer string=w158:string)  [unwired: 1 in]
              n26 = Insert Into Array(array=w155, new element=w158) -> (w154:string[])  [unwired: 1 in]
              n27 = Bundle By Name(cluster=w169, "Cycle Count"=w156) -> (w168:T3)
            }
            frame 1 {
              n28 = call "String Remove All Spaces.vi"("Input String"=w176) -> ("Spaces Removed"=w185:string)  [unwired: 13 in, 1 out]
              n29 = call "HexString to AsciiString.vi"("Hex String"=w185) -> ("ASCII String"=w181:string)  [unwired: 13 in, 1 out]
              n30 = Search and Replace String(replace all?=TRUE ("replace all? (F)"), input string=w181, search string="ÿ", replace string="") -> (result string=w178:string)  [unwired: 4 in, 3 out]
              n31 = Search and Replace String(replace all?=TRUE ("replace all? (F)"), input string=w178, search string="r", replace string="") -> (result string=w175:string)  [unwired: 4 in, 3 out]
              n32 = call "Build_ERD_Header_String_Array.vi"("ERD Name Array In"=w196, "ERD Number Array In"=w195, "ERD Name List"=w171, "New Header?"=w192, "ERD Number"=w191) -> ("ERD Name Array Out"=w194:string[], "ERD Number Array Out"=w193:string[])  [unwired: 13 in]
              n33 = Insert Into Array(array=w190, new element=w175) -> (w189:string[])  [unwired: 1 in]
              n34 = Bundle By Name(cluster=w201, "Model Number"=w175) -> (w200:T3)
            }
            frame 2 {
              n35 = call "String Remove All Spaces.vi"("Input String"=w206) -> ("Spaces Removed"=w219:string)  [unwired: 13 in, 1 out]
              n36 = call "HexString to AsciiString.vi"("Hex String"=w219) -> ("ASCII String"=w204:string)  [unwired: 13 in, 1 out]
              n37 = Search and Replace String(replace all?=TRUE ("replace all? (F)"), input string=w204, search string="ÿ", replace string="") -> (result string=w213:string)  [unwired: 4 in, 3 out]
              n38 = Search and Replace String(replace all?=TRUE ("replace all? (F)"), input string=w213, search string="r", replace string="") -> (result string=w207:string)  [unwired: 4 in, 3 out]
              n39 = Equal?(x=w204, y="\u0000\u0000\u0000\u0000\u0000\u0000\u0000\u0000\u0000\u0000\u0000\u0000\u0000\u0000\u0000\u0000\u0000\u0000\u0000\u0000\u0000\u0000\u0000\u0000\u0000\u0000\u0000\u0000\u0000\u0000\u0000\u0000") -> (x = y?=w209:bool)
              n40 = case shown="True" w209 {
                tunnel: [w236 "NO SERIAL NUMBER" ("y")] -> w208
                tunnel: w207 -> [w236 _]
                frame False {
                }
                frame True {
                }
              }
              n41 = call "Build_ERD_Header_String_Array.vi"("ERD Name Array In"=w230, "ERD Number Array In"=w229, "ERD Name List"=w202, "New Header?"=w226, "ERD Number"=w225) -> ("ERD Name Array Out"=w228:string[], "ERD Number Array Out"=w227:string[])  [unwired: 13 in]
              n42 = Insert Into Array(array=w224, new element=w208) -> (w223:string[])  [unwired: 1 in]
              n43 = Bundle By Name(cluster=w235, "Serial Number"=w208) -> (w234:T3)
            }
            frame 58 {
              n44 = call "VersionConversionData.vi"("Version In"=w239) -> ("Version Out"=w238:string)  [unwired: 9 in, 1 out]
              n45 = call "Build_ERD_Header_String_Array.vi"("ERD Name Array In"=w251, "ERD Number Array In"=w251, "ERD Name List"=w240, "New Header?"=w248, "ERD Number"=w247) -> ("ERD Name Array Out"=w250:string[], "ERD Number Array Out"=w249:string[])  [unwired: 13 in]
              n46 = Bundle By Name(cluster=w258, "Application Version"=w238) -> (w257:T2)
              n47 = Insert Into Array(array=w253, new element=w238) -> (w252:string[])  [unwired: 1 in]
            }
            frame 8202 {
              n48 = case shown="\"26\"" w264 {
                tunnel: ["Not Defined" "Basket Clean" "Drain & Spin" "Quick Rinse" "Bulky Items" "Sanitize" "Towels & Sheets" "Steam Refresh" "Normal/Mixed" "Whites" "Dark Colors" "Jeans" "Hand Wash" "Delicates" "Speed Wash" "Heavy Duty" "Allergen" "Power Clean" "Rinse & Spin" "Single Item" "Colors" "Cold Wash" "Water on Demand" "Deep Clean" "Cottons" "Easy Care" "Active Wear" "Timed Dry" "Dewrinkle" "Air Fluff" "Steam Refresh" "Steam Dewrinkle" "Speed Dry" "Mixed" "Quick Dry" "Casuals" "Warm Up" "Energy Saver"] -> w263
                frame "00", Default {
                }
                frame "01" {
                }
                frame "02" {
                }
                frame "03" {
                }
                frame "04" {
                }
                frame "05" {
                }
                frame "06" {
                }
                frame "07" {
                }
                frame "08" {
                }
                frame "09" {
                }
                frame "0A" {
                }
                frame "0B" {
                }
                frame "0C" {
                }
                frame "0D" {
                }
                frame "0E" {
                }
                frame "0F" {
                }
                frame "10" {
                }
                frame "11" {
                }
                frame "12" {
                }
                frame "13" {
                }
                frame "14" {
                }
                frame "15" {
                }
                frame "16" {
                }
                frame "26" {
                }
                frame "80" {
                }
                frame "81" {
                }
                frame "82" {
                }
                frame "83" {
                }
                frame "84" {
                }
                frame "85" {
                }
                frame "86" {
                }
                frame "87" {
                }
                frame "88" {
                }
                frame "89" {
                }
                frame "8A" {
                }
                frame "8B" {
                }
                frame "8C" {
                }
                frame "8D" {
                }
              }
              n49 = call "Build_ERD_Header_String_Array.vi"("ERD Name Array In"=w275, "ERD Number Array In"=w274, "ERD Name List"=w259, "New Header?"=w271, "ERD Number"=w270) -> ("ERD Name Array Out"=w273:string[], "ERD Number Array Out"=w272:string[])  [unwired: 13 in]
              n50 = Insert Into Array(array=w269, new element=w263) -> (w268:string[])  [unwired: 1 in]
              n51 = Bundle By Name(cluster=w280, "Cycle Name"=w263) -> (w279:T3)
            }
            frame 8208 {
              n52 = Decimal String To Number(string=w341) -> (number=w342:i32)  [unwired: 2 in, 1 out]
              n53 = To Unsigned Word Integer(number=w342) -> (unsigned 16bit integer=w331:u16)
              n54 = call "Build_ERD_Header_String_Array.vi"("ERD Name Array In"=w330, "ERD Number Array In"=w329, "ERD Name List"=w319, "New Header?"=w326, "ERD Number"=w325) -> ("ERD Name Array Out"=w328:string[], "ERD Number Array Out"=w327:string[])  [unwired: 13 in]
              n55 = Number To Decimal String(number=w331) -> (decimal integer string=w334:string)  [unwired: 1 in]
              n56 = Insert Into Array(array=w333, new element=w334) -> (w332:string[])  [unwired: 1 in]
              n57 = Bundle By Name(cluster=w340, "Delay Time"=w331) -> (w339:T3)
            }
            frame 8213 {
              n58 = case shown="\"05\"" w362 {
                selector: w362 -> [w365 _ _ _ _ _ _]
                tunnel: [w365 "EXTRA LIGHT" "LIGHT" "NORMAL" "HEAVY" "EXTRA HEAVY" "Disabled / Undefined"] -> w355
                frame Default {
                }
                frame "00" {
                }
                frame "01" {
                }
                frame "02" {
                }
                frame "03" {
                }
                frame "04" {
                }
                frame "05" {
                }
              }
              n59 = call "Build_ERD_Header_String_Array.vi"("ERD Name Array In"=w354, "ERD Number Array In"=w353, "ERD Name List"=w343, "New Header?"=w350, "ERD Number"=w349) -> ("ERD Name Array Out"=w352:string[], "ERD Number Array Out"=w351:string[])  [unwired: 13 in]
              n60 = Insert Into Array(array=w357, new element=w355) -> (w356:string[])  [unwired: 1 in]
              n61 = Bundle By Name(cluster=w364, "Soil Level"=w355) -> (w363:T3)
            }
            frame 61457 {
              n62 = call "Red_Micro_Parse.vi"("Data"=w391, "String Array In"=w380) -> ("Redundant Micro out"=w378:T6, "String Array Out"=w379:string[])  [unwired: 8 in]
              n63 = call "Build_ERD_Header_String_Array.vi"("ERD Name Array In"=w386, "ERD Number Array In"=w385, "ERD Name List"=w372, "New Header?"=w382, "ERD Number"=w381) -> ("ERD Name Array Out"=w384:string[], "ERD Number Array Out"=w383:string[])  [unwired: 13 in]
            }
            frame 59 {
              n64 = call "VersionConversionData.vi"("Version In"=w392) -> ("Version Out"=w393:string)  [unwired: 9 in, 1 out]
              n65 = call "Build_ERD_Header_String_Array.vi"("ERD Name Array In"=w406, "ERD Number Array In"=w405, "ERD Name List"=w394, "New Header?"=w402, "ERD Number"=w401) -> ("ERD Name Array Out"=w404:string[], "ERD Number Array Out"=w403:string[])  [unwired: 13 in]
              n66 = Bundle By Name(cluster=w413, "Parametric Version"=w393) -> (w412:T2)
              n67 = Insert Into Array(array=w408, new element=w393) -> (w407:string[])  [unwired: 1 in]
            }
            frame 64 {
              n68 = Decimal String To Number(string=w435) -> (number=w433:i32)  [unwired: 2 in, 1 out]
              n69 = To Unsigned Byte Integer(number=w433) -> (unsigned 8bit integer=w422:u8)
              n70 = Bundle By Name(cluster=w434, "Available Free Stack %"=w422) -> (w432:T3)
              n71 = Number To Decimal String(number=w422) -> (decimal integer string=w421:string)  [unwired: 1 in]
              n72 = call "Build_ERD_Header_String_Array.vi"("ERD Name Array In"=w428, "ERD Number Array In"=w427, "ERD Name List"=w414, "New Header?"=w424, "ERD Number"=w420) -> ("ERD Name Array Out"=w426:string[], "ERD Number Array Out"=w425:string[])  [unwired: 13 in]
              n73 = Insert Into Array(array=w430, new element=w421) -> (w423:string[])  [unwired: 1 in]
            }
            frame 61490 {
              n74 = call "HexStringToBoolean.vi"("Hex String"=w458) -> ("Boolean"=w450:bool)
              n75 = call "Build_ERD_Header_String_Array.vi"("ERD Name Array In"=w449, "ERD Number Array In"=w448, "ERD Name List"=w438, "New Header?"=w445, "ERD Number"=w444) -> ("ERD Name Array Out"=w447:string[], "ERD Number Array Out"=w446:string[])  [unwired: 13 in]
              n76 = case shown="True" w450 {
                tunnel: ["OFF" "ON"] -> w453
                frame False {
                }
                frame True {
                }
              }
              n77 = Insert Into Array(array=w452, new element=w453) -> (w451:string[])  [unwired: 1 in]
              n78 = Bundle By Name(cluster=w460, "Extra Rinse"=w450) -> (w459:T3)
            }
            frame 61491 {
              n79 = call "HexStringToBoolean.vi"("Hex String"=w483) -> ("Boolean"=w475:bool)
              n80 = call "Build_ERD_Header_String_Array.vi"("ERD Name Array In"=w474, "ERD Number Array In"=w473, "ERD Name List"=w463, "New Header?"=w470, "ERD Number"=w469) -> ("ERD Name Array Out"=w472:string[], "ERD Number Array Out"=w471:string[])  [unwired: 13 in]
              n81 = case shown="True" w475 {
                tunnel: ["OFF" "ON"] -> w478
                frame False {
                }
                frame True {
                }
              }
              n82 = Insert Into Array(array=w477, new element=w478) -> (w476:string[])  [unwired: 1 in]
              n83 = Bundle By Name(cluster=w485, "Deep Rinse / FS"=w475) -> (w484:T3)
            }
            frame 61492 {
              n84 = call "HexStringToBoolean.vi"("Hex String"=w508) -> ("Boolean"=w500:bool)
              n85 = call "Build_ERD_Header_String_Array.vi"("ERD Name Array In"=w499, "ERD Number Array In"=w498, "ERD Name List"=w488, "New Header?"=w495, "ERD Number"=w494) -> ("ERD Name Array Out"=w497:string[], "ERD Number Array Out"=w496:string[])  [unwired: 13 in]
              n86 = case shown="True" w500 {
                tunnel: ["OFF" "ON"] -> w503
                frame False {
                }
                frame True {
                }
              }
              n87 = Insert Into Array(array=w502, new element=w503) -> (w501:string[])  [unwired: 1 in]
              n88 = Bundle By Name(cluster=w510, "My Cycle"=w500) -> (w509:T3)
            }
            frame 61493 {
              n89 = case shown="\"04\"" w532 {
                selector: w532 -> [w535 _ _ _ _ _]
                tunnel: [w535 "NO SPIN" "NORMAL" "MORE " "MAX" "Disabled / Undefined"] -> w525
                frame Default {
                }
                frame "00" {
                }
                frame "01" {
                }
                frame "02" {
                }
                frame "03" {
                }
                frame "04" {
                }
              }
              n90 = call "Build_ERD_Header_String_Array.vi"("ERD Name Array In"=w524, "ERD Number Array In"=w523, "ERD Name List"=w513, "New Header?"=w520, "ERD Number"=w519) -> ("ERD Name Array Out"=w522:string[], "ERD Number Array Out"=w521:string[])  [unwired: 13 in]
              n91 = Insert Into Array(array=w527, new element=w525) -> (w526:string[])  [unwired: 1 in]
              n92 = Bundle By Name(cluster=w534, "Spin Level"=w525) -> (w533:T3)
            }
            frame 8228 {
              n93 = case shown="\"04\"" w560 {
                selector: w560 -> [w563 _ _ _ _ _ _]
                tunnel: [w563 "OFF" "TOMATO" "WINE" "BLOOD" "GRASS" "DIRT"] -> w547
                frame Default {
                }
                frame "00" {
                }
                frame "01" {
                }
                frame "02" {
                }
                frame "03" {
                }
                frame "04" {
                }
                frame "05" {
                }
              }
              n94 = call "Build_ERD_Header_String_Array.vi"("ERD Name Array In"=w555, "ERD Number Array In"=w554, "ERD Name List"=w541, "New Header?"=w551, "ERD Number"=w550) -> ("ERD Name Array Out"=w553:string[], "ERD Number Array Out"=w552:string[])  [unwired: 13 in]
              n95 = Insert Into Array(array=w549, new element=w547) -> (w548:string[])  [unwired: 1 in]
              n96 = Bundle By Name(cluster=w562, "Stain"=w547) -> (w561:T3)
            }
            frame 8379 {
              n97 = case shown="\"00\"" w590 {
                selector: w590 -> [w593 _ _ _ _ _ _ _]
                tunnel: [w593 "TAP COLD" "COLD" "COOL" "COLORS" "WARM" "HOT" "Disabled / Undefined"] -> w574
                frame Default {
                }
                frame "00" {
                }
                frame "01" {
                }
                frame "02" {
                }
                frame "03" {
                }
                frame "04" {
                }
                frame "05" {
                }
                frame "06" {
                }
              }
              n98 = Bundle By Name(cluster=w576, "User Temp Level"=w574) -> (w575:T8)
              n99 = call "Build_ERD_Header_String_Array.vi"("ERD Name Array In"=w585, "ERD Number Array In"=w584, "ERD Name List"=w570, "New Header?"=w579, "ERD Number"=w578) -> ("ERD Name Array Out"=w583:string[], "ERD Number Array Out"=w582:string[])  [unwired: 13 in]
              n100 = Insert Into Array(array=w581, new element=w574) -> (w580:string[])  [unwired: 1 in]
              n101 = Bundle By Name(cluster=w592, "Temp Level"=w574) -> (w591:T3)
            }
            frame 61496 {
              n102 = case shown="\"04\"" w622 {
                selector: w622 -> [w624 _ _ _ _ _]
                tunnel: [w624 "SMALL" "MEDIUM" "LARGE" "SUPER" "PRECISE FILL"] -> w604
                frame Default {
                }
                frame "00" {
                }
                frame "01" {
                }
                frame "02" {
                }
                frame "03" {
                }
                frame "04" {
                }
              }
              n103 = Bundle By Name(cluster=w606, "Load Size"=w604) -> (w605:T7)
              n104 = call "Build_ERD_Header_String_Array.vi"("ERD Name Array In"=w615, "ERD Number Array In"=w614, "ERD Name List"=string[] ["Load Size"], "New Header?"=w611, "ERD Number"=w610) -> ("ERD Name Array Out"=w613:string[], "ERD Number Array Out"=w612:string[])  [unwired: 13 in]
              n105 = Insert Into Array(array=w609, new element=w604) -> (w608:string[])  [unwired: 1 in]
              n106 = Bundle By Name(cluster=w623, "Load Size"=w604) -> (w621:T3)
            }
            frame 8192 {
              n107 = Decimal String To Number(string=w649) -> (number=w650:i32)  [unwired: 2 in, 1 out]
              n108 = case shown="3" w650 {
                tunnel: ["UNKOWN" ("Profile Status") "IDLE" ("Profile Status") "STANDBY" "RUN" "PAUSE" ("Profile Status") "ENDOFCYCLE" "DEMANDSIDEMANAGEMENTDELAYRUN" "DELAYRUN" "DELAY PAUSE" ("Profile Status") "DRAINTIMEOUT" "COMISSIONING" ("Profile Status") "BULKFLUSH" ("Profile Status") "BULK FLUSH" ("Profile Status")] -> w636
                frame 99, Default {
                }
                frame 0 {
                }
                frame 1 {
                }
                frame 2 {
                }
                frame 3 {
                }
                frame 4 {
                }
                frame 5 {
                }
                frame 6 {
                }
                frame 7 {
                }
                frame 8 {
                }
                frame 9 {
                }
                frame 10 {
                }
                frame 128 {
                }
              }
              n109 = call "Build_ERD_Header_String_Array.vi"("ERD Name Array In"=w644, "ERD Number Array In"=w643, "ERD Name List"=w630, "New Header?"=w640, "ERD Number"=w639) -> ("ERD Name Array Out"=w642:string[], "ERD Number Array Out"=w641:string[])  [unwired: 13 in]
              n110 = Insert Into Array(array=w638, new element=w636) -> (w637:string[])  [unwired: 1 in]
              n111 = Bundle By Name(cluster=w651, "Machine State"=w636) -> (w652:T3)
            }
            frame 61499 {
              n112 = Decimal String To Number(string=w685) -> (number=w688:i32)  [unwired: 2 in, 1 out]
              n113 = case shown="0, Default" w688 {
                tunnel: ["Cycle 0" ("Motor Profile") "Cycle 1" ("Motor Profile") "Cycle 2" ("Motor Profile") "Cycle 3" ("Motor Profile") "Cycle 4" ("Motor Profile") "Cycle 5" ("Motor Profile") "Cycle 6" ("Motor Profile") "Cycle 7" ("Motor Profile") "Cycle 8" ("Motor Profile") "Cycle 9" ("Motor Profile") "Cycle 10" ("Motor Profile") "Cycle 11" ("Motor Profile") "Cycle 12" ("Motor Profile") "Cycle 13" ("Motor Profile") "Cycle 14" ("Motor Profile") "Cycle 15" ("Motor Profile")] -> w678
                frame 0, Default {
                }
                frame 1 {
                }
                frame 2 {
                }
                frame 3 {
                }
                frame 4 {
                }
                frame 5 {
                }
                frame 6 {
                }
                frame 7 {
                }
                frame 8 {
                }
                frame 9 {
                }
                frame 10 {
                }
                frame 11 {
                }
                frame 12 {
                }
                frame 13 {
                }
                frame 14 {
                }
                frame 15 {
                }
              }
              n114 = call "Build_ERD_Header_String_Array.vi"("ERD Name Array In"=w677, "ERD Number Array In"=w676, "ERD Name List"=w666, "New Header?"=w673, "ERD Number"=w672) -> ("ERD Name Array Out"=w675:string[], "ERD Number Array Out"=w674:string[])  [unwired: 13 in]
              n115 = Insert Into Array(array=w680, new element=w678) -> (w679:string[])  [unwired: 1 in]
              n116 = Bundle By Name(cluster=w686, "Cycle Selected"=w678) -> (w687:T3)
            }
            frame 8232 {
              n117 = Decimal String To Number(string=w727) -> (number=w728:i32)  [unwired: 2 in, 1 out]
              n118 = To Unsigned Word Integer(number=w728) -> (unsigned 16bit integer=w717:u16)
              n119 = call "Build_ERD_Header_String_Array.vi"("ERD Name Array In"=w716, "ERD Number Array In"=w715, "ERD Name List"=w705, "New Header?"=w712, "ERD Number"=w711) -> ("ERD Name Array Out"=w714:string[], "ERD Number Array Out"=w713:string[])  [unwired: 13 in]
              n120 = Number To Decimal String(number=w717) -> (decimal integer string=w720:string)  [unwired: 1 in]
              n121 = Insert Into Array(array=w719, new element=w720) -> (w718:string[])  [unwired: 1 in]
              n122 = Bundle By Name(cluster=w726, "Soak Time"=w717) -> (w725:T3)
            }
            frame 61515 {
              n123 = call "Build_ERD_Header_String_Array.vi"("ERD Name Array In"=w740, "ERD Number Array In"=w739, "ERD Name List"=w729, "New Header?"=w734, "ERD Number"=w733) -> ("ERD Name Array Out"=w738:string[], "ERD Number Array Out"=w737:string[])  [unwired: 13 in]
              n124 = Insert Into Array(array=w743, new element=w741) -> (w742:string[])  [unwired: 1 in]
              n125 = Bundle By Name(cluster=w749, "Auto Soak Level"=w741) -> (w748:T3)
            }
            frame 61519 {
              n126 = case shown="\"00\", Default" w768 {
                tunnel: [FALSE ("Eco Wash") TRUE ("Eco Wash") TRUE ("Eco Wash")] -> w762
                frame "00", Default {
                }
                frame "01" {
                }
                frame "02" {
                }
              }
              n127 = case shown="True" w762 {
                tunnel: ["OFF" "ON"] -> w765
                frame False {
                }
                frame True {
                }
              }
              n128 = call "Build_ERD_Header_String_Array.vi"("ERD Name Array In"=w760, "ERD Number Array In"=w759, "ERD Name List"=string[] ["Deep Fill"], "New Header?"=w756, "ERD Number"=w755) -> ("ERD Name Array Out"=w758:string[], "ERD Number Array Out"=w757:string[])  [unwired: 13 in]
              n129 = Insert Into Array(array=w764, new element=w765) -> (w763:string[])  [unwired: 1 in]
              n130 = Bundle By Name(cluster=w772, "Deep Fill"=w762) -> (w771:T3)
            }
            frame 8229 {
              n131 = call "HexStringToBoolean.vi"("Hex String"=w800) -> ("Boolean"=w790:bool)
              n132 = case shown="True" w790 {
                tunnel: ["OFF" "ON"] -> w793
                frame False {
                }
                frame True {
                }
              }
              n133 = Insert Into Array(array=w792, new element=w793) -> (w791:string[])  [unwired: 1 in]
              n134 = call "Build_ERD_Header_String_Array.vi"("ERD Name Array In"=w788, "ERD Number Array In"=w787, "ERD Name List"=string[] ["Warm Rinse"], "New Header?"=w784, "ERD Number"=w783) -> ("ERD Name Array Out"=w786:string[], "ERD Number Array Out"=w785:string[])  [unwired: 13 in]
              n135 = Bundle By Name(cluster=w799, "Warm Rinse"=w790) -> (w798:T3)
            }
            frame 61537 {
              n136 = Decimal String To Number(string=w822) -> (number=w823:i32)  [unwired: 2 in, 1 out]
              n137 = To Unsigned Long Integer(number=w823) -> (unsigned 32bit integer=w815:u32)
              n138 = Bundle By Name(cluster=w821, "Remaining Cycle Time (s)"=w815) -> (w826:T3)
              n139 = Number To Decimal String(number=w815) -> (decimal integer string=w818:string)  [unwired: 1 in]
              n140 = call "Build_ERD_Header_String_Array.vi"("ERD Name Array In"=w813, "ERD Number Array In"=w812, "ERD Name List"=string[] ["Remaing Cycle Time"], "New Header?"=w809, "ERD Number"=w808) -> ("ERD Name Array Out"=w811:string[], "ERD Number Array Out"=w810:string[])  [unwired: 13 in]
              n141 = Insert Into Array(array=w817, new element=w818) -> (w816:string[])  [unwired: 1 in]
            }
            frame 61544 {
              n142 = call <vilib>:"Space Constant.vi"() -> ("String"=w832:string)
              n143 = Search and Replace String(replace all?=TRUE ("replace all? (F)"), input string=w827, search string=w832, replace string="" ("replace string (\"\")")) -> (result string=w830:string)  [unwired: 4 in, 3 out]
              n144 = Hexadecimal String To Number(string=w830) -> (number=w828:u32)  [unwired: 2 in, 1 out]
              n145 = Divide(x=w828, y=100.0) -> (x/y=w837:dbl)
              n146 = call "Build_ERD_Header_String_Array.vi"("ERD Name Array In"=w846, "ERD Number Array In"=w845, "ERD Name List"=string[] ["Wet Load Gallons"], "New Header?"=w842, "ERD Number"=w841) -> ("ERD Name Array Out"=w844:string[], "ERD Number Array Out"=w843:string[])  [unwired: 13 in]
              n147 = Bundle By Name(cluster=w839, "Wet Load Gal"=w837) -> (w838:T7)
              n148 = Number To Fractional String(number=w837) -> (F-format string=w850:string)  [unwired: 3 in]
              n149 = Insert Into Array(array=w849, new element=w850) -> (w848:string[])  [unwired: 1 in]
              n150 = Bundle By Name(cluster=w855, "Wet Load Gallons"=w837) -> (w854:T3)
            }
            frame 61545 {
              n151 = call <vilib>:"Space Constant.vi"() -> ("String"=w862:string)
              n152 = Search and Replace String(replace all?=TRUE ("replace all? (F)"), input string=w858, search string=w862, replace string="" ("replace string (\"\")")) -> (result string=w860:string)  [unwired: 4 in, 3 out]
              n153 = Hexadecimal String To Number(string=w860) -> (number=w857:u32)  [unwired: 2 in, 1 out]
              n154 = To Double Precision Float(number=w857) -> (double precision float=w885:dbl)
              n155 = Divide(x=w885, y=100.0) -> (x/y=w873:dbl)
              n156 = call "Build_ERD_Header_String_Array.vi"("ERD Name Array In"=w871, "ERD Number Array In"=w870, "ERD Name List"=string[] ["Tub Volume (Gal)"], "New Header?"=w867, "ERD Number"=w866) -> ("ERD Name Array Out"=w869:string[], "ERD Number Array Out"=w868:string[])  [unwired: 13 in]
              n157 = Bundle By Name(cluster=w884, "Tub Volume (Gal)"=w873) -> (w883:T3)
              n158 = Number To Fractional String(number=w873) -> (F-format string=w876:string)  [unwired: 3 in]
              n159 = Insert Into Array(array=w875, new element=w876) -> (w874:string[])  [unwired: 1 in]
            }
            frame 61546 {
              n160 = call <vilib>:"Space Constant.vi"() -> ("String"=w891:string)
              n161 = Search and Replace String(replace all?=TRUE ("replace all? (F)"), input string=w892, search string=w891, replace string="" ("replace string (\"\")")) -> (result string=w889:string)  [unwired: 4 in, 3 out]
              n162 = Hexadecimal String To Number(string=w889) -> (number=w888:u32)  [unwired: 2 in, 1 out]
              n163 = Divide(x=w888, y=1000.0) -> (x/y=w896:dbl)
              "x/y" <- w896
              n164 = call "Build_ERD_Header_String_Array.vi"("ERD Name Array In"=w905, "ERD Number Array In"=w904, "ERD Name List"=string[] ["Pressure (in H20)"], "New Header?"=w901, "ERD Number"=w900) -> ("ERD Name Array Out"=w903:string[], "ERD Number Array Out"=w902:string[])  [unwired: 13 in]
              n165 = Number To Fractional String(number=w896) -> (F-format string=w899:string)  [unwired: 3 in]
              n166 = Insert Into Array(array=w898, new element=w899) -> (w897:string[])  [unwired: 1 in]
              n167 = Bundle By Name(cluster=w914, "Pressure (inches H20)"=w896) -> (w913:T3)
            }
            frame 61549 {
              n168 = call <vilib>:"Space Constant.vi"() -> ("String"=w921:string)
              n169 = Search and Replace String(replace all?=TRUE ("replace all? (F)"), input string=w917, search string=w921, replace string="" ("replace string (\"\")")) -> (result string=w919:string)  [unwired: 4 in, 3 out]
              n170 = Hexadecimal String To Number(string=w919) -> (number=w918:u32)  [unwired: 2 in, 1 out]
              n171 = Divide(x=w918, y=100.0) -> (x/y=w925:dbl)
              n172 = Bundle By Name(cluster=w932, "Target Gallons"=w925) -> (w931:T8)
              n173 = Number To Fractional String(number=w925) -> (F-format string=w928:string)  [unwired: 3 in]
              n174 = Bundle By Name(cluster=w930, "Target Gallons"=w925) -> (w929:T7)
              n175 = call "Build_ERD_Header_String_Array.vi"("ERD Name Array In"=w938, "ERD Number Array In"=w937, "ERD Name List"=string[] ["Target Gallons"], "New Header?"=w934, "ERD Number"=w933) -> ("ERD Name Array Out"=w936:string[], "ERD Number Array Out"=w935:string[])  [unwired: 13 in]
              n176 = Insert Into Array(array=w927, new element=w928) -> (w926:string[])  [unwired: 1 in]
              n177 = Bundle By Name(cluster=w945, "Target Gallons"=w925) -> (w944:T3)
            }
            frame 61550 {
              n178 = case shown="\"11\"" w969 {
                selector: w969 -> [w970 _ _ _ _ _ _ _ _ _ _ _ _]
                tunnel: [w970 "UNKNOWN" "COTTON" "SYNTHETIC" "MIXED" "WET" "LOW FLOW" "SMALL" "MEDIUM" "LARGE" "SUPER" "SUPER PLUS" "MAX"] -> w950
                frame Default {
                }
                frame "0" {
                }
                frame "1" {
                }
                frame "2" {
                }
                frame "3" {
                }
                frame "4" {
                }
                frame "5" {
                }
                frame "6" {
                }
                frame "7" {
                }
                frame "8" {
                }
                frame "9" {
                }
                frame "10" {
                }
                frame "11" {
                }
              }
              n179 = call "Build_ERD_Header_String_Array.vi"("ERD Name Array In"=w961, "ERD Number Array In"=w959, "ERD Name List"=string[] ["Load Type"], "New Header?"=w956, "ERD Number"=w955) -> ("ERD Name Array Out"=w958:string[], "ERD Number Array Out"=w957:string[])  [unwired: 13 in]
              n180 = Bundle By Name(cluster=w954, "Load Type"=w950) -> (w953:T7)
              n181 = Insert Into Array(array=w951, new element=w950) -> (w952:string[])  [unwired: 1 in]
              n182 = Bundle By Name(cluster=w968, "Load Type"=w950) -> (w967:T3)
            }
            frame 61551 {
              n183 = call "HexStringToBoolean.vi"("Hex String"=w1004) -> ("Boolean"=w993:bool)
              n184 = case shown="True" w993 {
                tunnel: ["OFF" "ON"] -> w996
                frame False {
                }
                frame True {
                }
              }
              n185 = call "Build_ERD_Header_String_Array.vi"("ERD Name Array In"=w991, "ERD Number Array In"=w990, "ERD Name List"=string[] ["Lid Switch"], "New Header?"=w987, "ERD Number"=w986) -> ("ERD Name Array Out"=w989:string[], "ERD Number Array Out"=w988:string[])  [unwired: 13 in]
              n186 = Insert Into Array(array=w995, new element=w996) -> (w994:string[])  [unwired: 1 in]
              n187 = Bundle By Name(cluster=w1005, "Lid Switch"=w993) -> (w1003:T3)
            }
            frame 61554 {
              n188 = String Subset(string=w1030, offset (0)=3, length (rest)=2 ("length (rest)")) -> (substring=w1031:string)
              n189 = Hexadecimal String To Number(string=w1031) -> (number=w1029:u32)  [unwired: 2 in, 1 out]
              n190 = case shown="0, Default" w1029 {
                tunnel: ["UNLOCKED" "LOCKED" "FAILURE"] -> w1013
                frame 0, Default {
                }
                frame 1 {
                }
                frame 2 {
                }
              }
              n191 = call "Build_ERD_Header_String_Array.vi"("ERD Name Array In"=w1019, "ERD Number Array In"=w1018, "ERD Name List"=string[] ["Lid Lock Req State"], "New Header?"=w1012, "ERD Number"=w1011) -> ("ERD Name Array Out"=w1017:string[], "ERD Number Array Out"=w1016:string[])  [unwired: 13 in]
              n192 = Insert Into Array(array=w1015, new element=w1013) -> (w1014:string[])  [unwired: 1 in]
              n193 = Bundle By Name(cluster=w1026, "Lid Lock Req State"=w1013) -> (w1025:T3)
            }
            frame 61555 {
              n194 = Decimal String To Number(string=w1058) -> (number=w1059:i32)  [unwired: 2 in, 1 out]
              n195 = case shown="2" w1059 {
                tunnel: ["Unlocked" ("Motor Profile") "Locked" ("Motor Profile") "Failure" ("Motor Profile")] -> w1040
                frame 0, Default {
                }
                frame 1 {
                }
                frame 2 {
                }
              }
              n196 = call "Build_ERD_Header_String_Array.vi"("ERD Name Array In"=w1048, "ERD Number Array In"=w1047, "ERD Name List"=string[] ["Lid Lock Status"], "New Header?"=w1044, "ERD Number"=w1043) -> ("ERD Name Array Out"=w1046:string[], "ERD Number Array Out"=w1045:string[])  [unwired: 13 in]
              n197 = Insert Into Array(array=w1042, new element=w1040) -> (w1041:string[])  [unwired: 1 in]
              n198 = Bundle By Name(cluster=w1057, "Lid Lock Status"=w1040) -> (w1056:T3)
            }
            frame 61556 {
              n199 = String Subset(string=w1084, offset (0)=3, length (rest)=2 ("length (rest)")) -> (substring=w1087:string)
              n200 = String Subset(string=w1084, offset (0)=0, length (rest)=2 ("length (rest)")) -> (substring=w1090:string)
              n201 = Hexadecimal String To Number(string=w1090) -> (number=w1089:u32)  [unwired: 2 in, 1 out]
              n202 = Hexadecimal String To Number(string=w1087) -> (number=w1086:u32)  [unwired: 2 in, 1 out]
              n203 = case shown="0, Default" w1086 {
                tunnel: ["Unknown" "Started" "Stopped" "Paused" "Resumed" "Selected" "Completed"] -> w1067
                frame 0, Default {
                }
                frame 6 {
                }
                frame 7 {
                }
                frame 8 {
                }
                frame 9 {
                }
                frame 10 {
                }
                frame 11 {
                }
              }
              n204 = Number To Decimal String(number=w1089) -> (decimal integer string=w1088:string)  [unwired: 1 in]
              n205 = call "Build_ERD_Header_String_Array.vi"("ERD Name Array In"=w1075, "ERD Number Array In"=w1074, "ERD Name List"=string[] ["Cycle Engine State"], "New Header?"=w1071, "ERD Number"=w1070) -> ("ERD Name Array Out"=w1073:string[], "ERD Number Array Out"=w1072:string[])  [unwired: 13 in]
              n206 = call <vilib>:"Space Constant.vi"() -> ("String"=w1085:string)
              n207 = Concatenate Strings("Cycle" ("string"), w1085, w1088, w1085, w1067) -> (w1066:string)
              n208 = Bundle By Name(cluster=w1096, "Cycle Engine State"=w1066) -> (w1095:T3)
              n209 = Insert Into Array(array=w1069, new element=w1066) -> (w1068:string[])  [unwired: 1 in]
            }
            frame 61559 {
              n210 = call <vilib>:"Space Constant.vi"() -> ("String"=w1109:string)
              n211 = Search and Replace String(replace all?=TRUE ("replace all? (F)"), input string=w1104, search string=w1109, replace string="" ("replace string (\"\")")) -> (result string=w1107:string)  [unwired: 4 in, 3 out]
              n212 = Hexadecimal String To Number(string=w1107) -> (number=w1105:u32)  [unwired: 2 in, 1 out]
              n213 = Divide(x=w1105, y=10.0) -> (x/y=w1120:dbl)
              n214 = Bundle By Name(cluster=w1125, "Current Water Temp"=w1120) -> (w1124:T8)
              n215 = Bundle By Name(cluster=w1132, "Temperature (F)"=w1120) -> (w1131:T3)
              n216 = Number To Fractional String(number=w1120) -> (F-format string=w1123:string)  [unwired: 3 in]
              n217 = call "Build_ERD_Header_String_Array.vi"("ERD Name Array In"=w1118, "ERD Number Array In"=w1117, "ERD Name List"=string[] ["Temperature"], "New Header?"=w1114, "ERD Number"=w1113) -> ("ERD Name Array Out"=w1116:string[], "ERD Number Array Out"=w1115:string[])  [unwired: 13 in]
              n218 = Insert Into Array(array=w1122, new element=w1123) -> (w1121:string[])  [unwired: 1 in]
            }
            frame 61561 {
              n219 = String Subset(string=w1156, offset (0)=3, length (rest)=2 ("length (rest)")) -> (substring=w1157:string)
              n220 = call "HexStringToBoolean.vi"("Hex String"=w1157) -> ("Boolean"=w1143:bool)
              n221 = call "Build_ERD_Header_String_Array.vi"("ERD Name Array In"=w1149, "ERD Number Array In"=w1148, "ERD Name List"=string[] ["Recirc. Pump"], "New Header?"=w1145, "ERD Number"=w1144) -> ("ERD Name Array Out"=w1147:string[], "ERD Number Array Out"=w1146:string[])  [unwired: 13 in]
              n222 = case shown="True" w1143 {
                tunnel: ["OFF" "ON"] -> w1137
                frame False {
                }
                frame True {
                }
              }
              n223 = Insert Into Array(array=w1139, new element=w1137) -> (w1138:string[])  [unwired: 1 in]
              n224 = Bundle By Name(cluster=w1155, "Recirc. Pump"=w1143) -> (w1154:T3)
            }
            frame 61563 {
              n225 = case shown="\"00\"" w1182 {
                selector: w1182 -> [w1184 _ _ _ _ _ _]
                tunnel: [w1184 "NONE" "FILL" "SOAK" "WASH" "RINSE" "SPIN"] -> w1172
                frame Default {
                }
                frame "00" {
                }
                frame "01" {
                }
                frame "02" {
                }
                frame "04" {
                }
                frame "08" {
                }
                frame "10" {
                }
              }
              n226 = call "Build_ERD_Header_String_Array.vi"("ERD Name Array In"=w1170, "ERD Number Array In"=w1169, "ERD Name List"=string[] ["Sub-Cycle"], "New Header?"=w1166, "ERD Number"=w1165) -> ("ERD Name Array Out"=w1168:string[], "ERD Number Array Out"=w1167:string[])  [unwired: 13 in]
              n227 = Insert Into Array(array=w1174, new element=w1172) -> (w1173:string[])  [unwired: 1 in]
              n228 = Bundle By Name(cluster=w1183, "Sub-Cycle"=w1172) -> (w1181:T3)
            }
            frame 61565 {
              n229 = call <vilib>:"Space Constant.vi"() -> ("String"=w1196:string)
              n230 = Search and Replace String(replace all?=TRUE ("replace all? (F)"), input string=w1192, search string=w1196, replace string="" ("replace string (\"\")")) -> (result string=w1194:string)  [unwired: 4 in, 3 out]
              n231 = Hexadecimal String To Number(string=w1194) -> (number=w1191:u32)  [unwired: 2 in, 1 out]
              n232 = Divide(x=w1191, y=100.0) -> (x/y=w1220:dbl)
              n233 = Bundle By Name(cluster=w1204, "Target Level"=w1220) -> (w1203:T8)
              n234 = call "Build_ERD_Header_String_Array.vi"("ERD Name Array In"=w1210, "ERD Number Array In"=w1209, "ERD Name List"=string[] ["Target Level (in)"], "New Header?"=w1206, "ERD Number"=w1205) -> ("ERD Name Array Out"=w1208:string[], "ERD Number Array Out"=w1207:string[])  [unwired: 13 in]
              n235 = Number To Decimal String(number=w1220) -> (decimal integer string=w1202:string)  [unwired: 1 in]
              n236 = Insert Into Array(array=w1201, new element=w1202) -> (w1200:string[])  [unwired: 1 in]
              n237 = Bundle By Name(cluster=w1218, "Target Level (inches)"=w1220) -> (w1217:T3)
            }
            frame 61568 {
              n238 = case shown="\"01\"" w1242 {
                selector: w1242 -> [w1243 _ _]
                tunnel: [w1243 "LOCKED" ("Motor Profile") "UNLOCKED" ("Motor Profile")] -> w1231
                frame "0", Default {
                }
                frame "00" {
                }
                frame "01" {
                }
              }
              n239 = call "Build_ERD_Header_String_Array.vi"("ERD Name Array In"=w1229, "ERD Number Array In"=w1228, "ERD Name List"=string[] ["Lid Lock FB"], "New Header?"=w1225, "ERD Number"=w1224) -> ("ERD Name Array Out"=w1227:string[], "ERD Number Array Out"=w1226:string[])  [unwired: 13 in]
              n240 = Insert Into Array(array=w1233, new element=w1231) -> (w1232:string[])  [unwired: 1 in]
              n241 = Bundle By Name(cluster=w1241, "Lid Lock FB"=w1231) -> (w1240:T3)
            }
            frame 61570 {
              (unwired) 10.0 ("y")
              n242 = call <vilib>:"Space Constant.vi"() -> ("String"=w1251:string)
              n243 = Search and Replace String(replace all?=TRUE ("replace all? (F)"), input string=w1246, search string=w1251, replace string="" ("replace string (\"\")")) -> (result string=w1249:string)  [unwired: 4 in, 3 out]
              n244 = Hexadecimal String To Number(string=w1249) -> (number=w1247:u32)  [unwired: 2 in, 1 out]
              n245 = To Double Precision Float(number=w1247) -> (double precision float=w1275:dbl)
              n246 = Divide(x=w1275, y=10.0) -> (x/y=w1255:dbl)
              n247 = call "Build_ERD_Header_String_Array.vi"("ERD Name Array In"=w1266, "ERD Number Array In"=w1265, "ERD Name List"=string[] ["Target Bath Temp (F)"], "New Header?"=w1262, "ERD Number"=w1261) -> ("ERD Name Array Out"=w1264:string[], "ERD Number Array Out"=w1263:string[])  [unwired: 13 in]
              n248 = Bundle By Name(cluster=w1260, "Target Bath Temp"=w1255) -> (w1259:T8)
              n249 = Number To Fractional String(number=w1255) -> (F-format string=w1256:string)  [unwired: 3 in]
              n250 = Insert Into Array(array=w1258, new element=w1256) -> (w1257:string[])  [unwired: 1 in]
              n251 = Bundle By Name(cluster=w1274, "Target Bath Temp (F)"=w1255) -> (w1273:T3)
            }
            frame 61571 {
              n252 = Decimal String To Number(string=w1300) -> (number=w1301:i32)  [unwired: 2 in, 1 out]
              n253 = To Double Precision Float(number=w1301) -> (double precision float=w1303:dbl)
              n254 = Divide(x=w1303, y=10.0) -> (x/y=w1282:dbl)
              n255 = Bundle By Name(cluster=w1292, "Current Bath Temp"=w1282) -> (w1291:T8)
              n256 = call "Build_ERD_Header_String_Array.vi"("ERD Name Array In"=w1289, "ERD Number Array In"=w1288, "ERD Name List"=string[] ["Current Bath Temp (F)"], "New Header?"=w1281, "ERD Number"=w1280) -> ("ERD Name Array Out"=w1287:string[], "ERD Number Array Out"=w1286:string[])  [unwired: 13 in]
              n257 = Number To Fractional String(number=w1282) -> (F-format string=w1285:string)  [unwired: 3 in]
              n258 = Insert Into Array(array=w1284, new element=w1285) -> (w1283:string[])  [unwired: 1 in]
              n259 = Bundle By Name(cluster=w1299, "Current Bath Temp (F)"=w1282) -> (w1298:T3)
            }
            frame 61572 {
              n260 = call <vilib>:"Space Constant.vi"() -> ("String"=w1309:string)
              n261 = Search and Replace String(replace all?=TRUE ("replace all? (F)"), input string=w1304, search string=w1309, replace string="" ("replace string (\"\")")) -> (result string=w1307:string)  [unwired: 4 in, 3 out]
              n262 = Hexadecimal String To Number(string=w1307) -> (number=w1305:u32)  [unwired: 2 in, 1 out]
              n263 = Divide(x=w1305, y=10.0) -> (x/y=w1315:dbl)
              n264 = Number To Fractional String(number=w1315) -> (F-format string=w1318:string)  [unwired: 3 in]
              n265 = Insert Into Array(array=w1317, new element=w1318) -> (w1316:string[])  [unwired: 1 in]
              n266 = call "Build_ERD_Header_String_Array.vi"("ERD Name Array In"=w1324, "ERD Number Array In"=w1323, "ERD Name List"=string[] ["Cold Inlet Temp (F)"], "New Header?"=w1314, "ERD Number"=w1313) -> ("ERD Name Array Out"=w1322:string[], "ERD Number Array Out"=w1321:string[])  [unwired: 13 in]
              n267 = Bundle By Name(cluster=w1320, "Cold Inlet Temp"=w1315) -> (w1319:T8)
            }
            frame 61573 {
              n268 = call <vilib>:"Space Constant.vi"() -> ("String"=w1338:string)
              n269 = Search and Replace String(replace all?=TRUE ("replace all? (F)"), input string=w1333, search string=w1338, replace string="" ("replace string (\"\")")) -> (result string=w1336:string)  [unwired: 4 in, 3 out]
              n270 = Hexadecimal String To Number(string=w1336) -> (number=w1334:u32)  [unwired: 2 in, 1 out]
              n271 = Divide(x=w1334, y=10.0) -> (x/y=w1349:dbl)
              n272 = Number To Fractional String(number=w1349) -> (F-format string=w1354:string)  [unwired: 3 in]
              n273 = Insert Into Array(array=w1353, new element=w1354) -> (w1352:string[])  [unwired: 1 in]
              n274 = call "Build_ERD_Header_String_Array.vi"("ERD Name Array In"=w1347, "ERD Number Array In"=w1346, "ERD Name List"=string[] ["Hot Inlet temp (F)"], "New Header?"=w1343, "ERD Number"=w1342) -> ("ERD Name Array Out"=w1345:string[], "ERD Number Array Out"=w1344:string[])  [unwired: 13 in]
              n275 = Bundle By Name(cluster=w1351, "Hot Inlet Temp"=w1349) -> (w1350:T8)
            }
            frame 61574 {
              n276 = Decimal String To Number(string=w1382) -> (number=w1383:i32)  [unwired: 2 in, 1 out]
              n277 = To Double Precision Float(number=w1383) -> (double precision float=w1384:dbl)
              n278 = Divide(x=w1384, y=10.0) -> (x/y=w1365:dbl)
              n279 = call "Build_ERD_Header_String_Array.vi"("ERD Name Array In"=w1376, "ERD Number Array In"=w1375, "ERD Name List"=string[] ["Warm Inlet Temp (F)"], "New Header?"=w1372, "ERD Number"=w1371) -> ("ERD Name Array Out"=w1374:string[], "ERD Number Array Out"=w1373:string[])  [unwired: 13 in]
              n280 = Bundle By Name(cluster=w1370, "Warm Inlet Temp"=w1365) -> (w1369:T8)
              n281 = Number To Fractional String(number=w1365) -> (F-format string=w1368:string)  [unwired: 3 in]
              n282 = Insert Into Array(array=w1367, new element=w1368) -> (w1366:string[])  [unwired: 1 in]
            }
            frame 61575 {
              n283 = String Subset(string=w1411, offset (0)=0, length (rest)=2 ("length (rest)")) -> (substring=w1427:string)
              n284 = String Subset(string=w1411, offset (0)=3, length (rest)=2 ("length (rest)")) -> (substring=w1426:string)
              n285 = String Subset(string=w1411, offset (0)=6, length (rest)=2 ("length (rest)")) -> (substring=w1416:string)
              n286 = String Subset(string=w1411, offset (0)=9, length (rest)=2 ("length (rest)")) -> (substring=w1417:string)
              n287 = Concatenate Strings(w1427, w1426) -> (w1425:string)
              n288 = Concatenate Strings(w1416, w1417) -> (w1418:string)
              n289 = Hexadecimal String To Number(string=w1425) -> (number=w1422:u32)  [unwired: 2 in, 1 out]
              n290 = Hexadecimal String To Number(string=w1418) -> (number=w1421:u32)  [unwired: 2 in, 1 out]
              n291 = To Double Precision Float(number=w1422) -> (double precision float=w1423:dbl)
              n292 = To Double Precision Float(number=w1421) -> (double precision float=w1420:dbl)
              n293 = Divide(x=w1423, y=100.0) -> (x/y=w1397:dbl)
              n294 = Divide(x=w1420, y=100.0) -> (x/y=w1396:dbl)
              n295 = Bundle By Name(cluster=w1405, "Cold Gallons"=w1396) -> (w1404:T8)
              n296 = call "Build_ERD_Header_String_Array.vi"("ERD Name Array In"=w1402, "ERD Number Array In"=w1401, "ERD Name List"=string[] ["Hot Gallons", "Cold Gallons"], "New Header?"=w1392, "ERD Number"=w1391) -> ("ERD Name Array Out"=w1400:string[], "ERD Number Array Out"=w1399:string[])  [unwired: 13 in]
              n297 = Bundle By Name(cluster=w1404, "Hot Gallons"=w1397) -> (w1406:T8)
              n298 = Number To Fractional String(number=w1397) -> (F-format string=w1398:string)  [unwired: 3 in]
              n299 = Number To Fractional String(number=w1396) -> (F-format string=w1395:string)  [unwired: 3 in]
              n300 = Insert Into Array(array=w1394, new element #1=w1398, new element #2=w1395) -> (w1393:string[])  [unwired: 1 in]
            }
            frame 61576 {
              n301 = String Subset(string=w1459, offset (0)=0, length (rest)=2 ("length (rest)")) -> (substring=w1469:string)
              n302 = String Subset(string=w1459, offset (0)=3, length (rest)=2 ("length (rest)")) -> (substring=w1468:string)
              n303 = String Subset(string=w1459, offset (0)=6, length (rest)=2 ("length (rest)")) -> (substring=w1464:string)
              n304 = String Subset(string=w1459, offset (0)=9, length (rest)=2 ("length (rest)")) -> (substring=w1465:string)
              n305 = Concatenate Strings(w1469, w1468) -> (w1467:string)
              n306 = Concatenate Strings(w1464, w1465) -> (w1466:string)
              n307 = Hexadecimal String To Number(string=w1467) -> (number=w1458:u32)  [unwired: 2 in, 1 out]
              n308 = Hexadecimal String To Number(string=w1466) -> (number=w1457:u32)  [unwired: 2 in, 1 out]
              n309 = To Unsigned Word Integer(number=w1458) -> (unsigned 16bit integer=w1438:u16)
              n310 = To Unsigned Word Integer(number=w1457) -> (unsigned 16bit integer=w1437:u16)
              n311 = Bundle By Name(cluster=w1444, "Cold Seg Valve Time"=w1437) -> (w1443:T8)
              n312 = call "Build_ERD_Header_String_Array.vi"("ERD Name Array In"=w1451, "ERD Number Array In"=w1450, "ERD Name List"=string[] ["Hot Seg Valve Time (s)", "Cold Seg Valve Time (s)"], "New Header?"=w1447, "ERD Number"=w1446) -> ("ERD Name Array Out"=w1449:string[], "ERD Number Array Out"=w1448:string[])  [unwired: 13 in]
              n313 = Bundle By Name(cluster=w1443, "Hot Seg Valve Time"=w1438) -> (w1445:T8)
              n314 = Number To Decimal String(number=w1438) -> (decimal integer string=w1442:string)  [unwired: 1 in]
              n315 = Number To Decimal String(number=w1437) -> (decimal integer string=w1439:string)  [unwired: 1 in]
              n316 = Insert Into Array(array=w1441, new element #1=w1442, new element #2=w1439) -> (w1440:string[])  [unwired: 1 in]
            }
            frame 61577 {
              n317 = call "HexStringToBoolean.vi"("Hex String"=w1495) -> ("Boolean"=w1479:bool)
              n318 = Bundle By Name(cluster=w1496, "Child Safety"=w1479) -> (w1494:T3)
              n319 = call "Build_ERD_Header_String_Array.vi"("ERD Name Array In"=w1488, "ERD Number Array In"=w1487, "ERD Name List"=string[] ["Child Safety"], "New Header?"=w1484, "ERD Number"=w1483) -> ("ERD Name Array Out"=w1486:string[], "ERD Number Array Out"=w1485:string[])  [unwired: 13 in]
              n320 = case shown="True" w1479 {
                tunnel: ["OFF" "ON"] -> w1482
                frame False {
                }
                frame True {
                }
              }
              n321 = Insert Into Array(array=w1481, new element=w1482) -> (w1480:string[])  [unwired: 1 in]
            }
            frame 61578 {
              n322 = call <vilib>:"Space Constant.vi"() -> ("String"=w1506:string)
              n323 = Search and Replace String(replace all?=TRUE ("replace all? (F)"), input string=w1502, search string=w1506, replace string="" ("replace string (\"\")")) -> (result string=w1504:string)  [unwired: 4 in, 3 out]
              n324 = Hexadecimal String To Number(string=w1504) -> (number=w1501:u32)  [unwired: 2 in, 1 out]
              n325 = Divide(x=w1501, y=100.0) -> (x/y=w1512:dbl)
              n326 = call "Build_ERD_Header_String_Array.vi"("ERD Name Array In"=w1521, "ERD Number Array In"=w1520, "ERD Name List"=string[] ["Segment Gallons"], "New Header?"=w1511, "ERD Number"=w1510) -> ("ERD Name Array Out"=w1519:string[], "ERD Number Array Out"=w1518:string[])  [unwired: 13 in]
              n327 = Bundle By Name(cluster=w1517, "Segment Gallons"=w1512) -> (w1516:T8)
              n328 = Number To Fractional String(number=w1512) -> (F-format string=w1515:string)  [unwired: 3 in]
              n329 = Insert Into Array(array=w1514, new element=w1515) -> (w1513:string[])  [unwired: 1 in]
            }
            frame 61594 {
              n330 = call "HexStringToBoolean.vi"("Hex String"=w1552) -> ("Boolean"=w1539:bool)
              n331 = call "Build_ERD_Header_String_Array.vi"("ERD Name Array In"=w1545, "ERD Number Array In"=w1544, "ERD Name List"=string[] ["Drain Pump"], "New Header?"=w1541, "ERD Number"=w1540) -> ("ERD Name Array Out"=w1543:string[], "ERD Number Array Out"=w1542:string[])  [unwired: 13 in]
              n332 = case shown="True" w1539 {
                tunnel: ["OFF" "ON"] -> w1536
                frame False {
                }
                frame True {
                }
              }
              n333 = Insert Into Array(array=w1538, new element=w1536) -> (w1537:string[])  [unwired: 1 in]
              n334 = Bundle By Name(cluster=w1551, "Drain Pump"=w1539) -> (w1550:T3)
            }
            frame 61595 {
              n335 = call "HexStringToBoolean.vi"("Hex String"=w1575) -> ("Boolean"=w1560:bool)
              n336 = call "Build_ERD_Header_String_Array.vi"("ERD Name Array In"=w1567, "ERD Number Array In"=w1566, "ERD Name List"=string[] ["Valve Relay"], "New Header?"=w1559, "ERD Number"=w1558) -> ("ERD Name Array Out"=w1565:string[], "ERD Number Array Out"=w1564:string[])  [unwired: 13 in]
              n337 = case shown="True" w1560 {
                tunnel: ["OFF" "ON"] -> w1563
                frame False {
                }
                frame True {
                }
              }
              n338 = Insert Into Array(array=w1562, new element=w1563) -> (w1561:string[])  [unwired: 1 in]
              n339 = Bundle By Name(cluster=w1577, "Valve Relay"=w1560) -> (w1576:T3)
            }
            frame 61596 {
              n340 = Decimal String To Number(string=w1604) -> (number=w1609:i32)  [unwired: 2 in, 1 out]
              n341 = Number To Boolean Array(number=w1609) -> (Boolean array=w1589:bool[])
              n342 = for {
                N: 5 -> [_]
                tunnel: w1589 -> [w1611] mode=indexing
                tunnel: [w1610] -> w1588 mode=indexing
                n343 = case shown="True" w1611 {
                  tunnel: ["OFF" "ON"] -> w1610
                  frame False {
                  }
                  frame True {
                  }
                }
              }
              n344 = Index Array(array=w1589) -> (element #1=w1606:bool, element #2=w1605:bool, element #3=w1601:bool, element #4=w1600:bool, element #5=w1583:bool)  [unwired: 5 in]
              n345 = call "Build_ERD_Header_String_Array.vi"("ERD Name Array In"=w1597, "ERD Number Array In"=w1596, "ERD Name List"=string[] ["Hot Valve", "Cold Valve", "Spray Valve", "Fab Soft Valve", "Bulk Disp Valve"], "New Header?"=w1593, "ERD Number"=w1592) -> ("ERD Name Array Out"=w1595:string[], "ERD Number Array Out"=w1594:string[])  [unwired: 13 in]
              n346 = Bundle By Name(cluster=w1608, "Hot  Water Valve"=w1606, "Cold Water Valve"=w1605, "Spray/Rinse Valve"=w1601, "Fabric Soft Valve"=w1600, "Bulk Disp Valve"=w1583) -> (w1607:T3)
              n347 = Insert Into Array(array=w1591, new element=w1588) -> (w1590:string[])  [unwired: 1 in]
            }
            frame 61598 {
              n348 = call <vilib>:"Space Constant.vi"() -> ("String"=w1619:string)
              n349 = Search and Replace String(replace all?=TRUE ("replace all? (F)"), input string=w1614, search string=w1619, replace string="" ("replace string (\"\")")) -> (result string=w1617:string)  [unwired: 4 in, 3 out]
              n350 = Hexadecimal String To Number(string=w1617) -> (number=w1615:u32)  [unwired: 2 in, 1 out]
              n351 = Divide(x=w1615, y=1024.0) -> (x/y=w1630:dbl)
              n352 = Bundle By Name(cluster=w1635, "Ramp Avg Current"=w1630) -> (w1634:T7)
              n353 = call "Build_ERD_Header_String_Array.vi"("ERD Name Array In"=w1628, "ERD Number Array In"=w1627, "ERD Name List"=string[] ["Ramp Avg Current"], "New Header?"=w1624, "ERD Number"=w1623) -> ("ERD Name Array Out"=w1626:string[], "ERD Number Array Out"=w1625:string[])  [unwired: 13 in]
              n354 = Number To Fractional String(number=w1630) -> (F-format string=w1633:string)  [unwired: 3 in]
              n355 = Insert Into Array(array=w1632, new element=w1633) -> (w1631:string[])  [unwired: 1 in]
            }
            frame 61599 {
              n356 = call <vilib>:"Space Constant.vi"() -> ("String"=w1648:string)
              n357 = Search and Replace String(replace all?=TRUE ("replace all? (F)"), input string=w1644, search string=w1648, replace string="" ("replace string (\"\")")) -> (result string=w1646:string)  [unwired: 4 in, 3 out]
              n358 = Hexadecimal String To Number(string=w1646) -> (number=w1643:u32)  [unwired: 2 in, 1 out]
              n359 = Divide(x=w1643, y=32.0) -> (x/y=w1659:dbl)
              n360 = call "Build_ERD_Header_String_Array.vi"("ERD Name Array In"=w1657, "ERD Number Array In"=w1656, "ERD Name List"=string[] ["Coast Line Voltage"], "New Header?"=w1653, "ERD Number"=w1652) -> ("ERD Name Array Out"=w1655:string[], "ERD Number Array Out"=w1654:string[])  [unwired: 13 in]
              n361 = Bundle By Name(cluster=w1664, "Coast Line Voltage"=w1659) -> (w1663:T7)
              n362 = Number To Fractional String(number=w1659) -> (F-format string=w1662:string)  [unwired: 3 in]
              n363 = Insert Into Array(array=w1661, new element=w1662) -> (w1660:string[])  [unwired: 1 in]
            }
            frame 61600 {
              n364 = Decimal String To Number(string=w1691) -> (number=w1692:i32)  [unwired: 2 in, 1 out]
              n365 = To Unsigned Word Integer(number=w1692) -> (unsigned 16bit integer=w1682:u16)
              n366 = Bundle By Name(cluster=w1687, "Ramp  Speed"=w1682) -> (w1686:T7)
              n367 = Number To Decimal String(number=w1682) -> (decimal integer string=w1685:string)  [unwired: 1 in]
              n368 = call "Build_ERD_Header_String_Array.vi"("ERD Name Array In"=w1680, "ERD Number Array In"=w1679, "ERD Name List"=string[] ["Ramp Speed"], "New Header?"=w1676, "ERD Number"=w1675) -> ("ERD Name Array Out"=w1678:string[], "ERD Number Array Out"=w1677:string[])  [unwired: 13 in]
              n369 = Insert Into Array(array=w1684, new element=w1685) -> (w1683:string[])  [unwired: 1 in]
            }
            frame 61601 {
              n370 = Decimal String To Number(string=w1715) -> (number=w1716:i32)  [unwired: 2 in, 1 out]
              n371 = To Unsigned Word Integer(number=w1716) -> (unsigned 16bit integer=w1699:u16)
              n372 = Bundle By Name(cluster=w1704, "Ramp Time"=w1699) -> (w1703:T7)
              n373 = Number To Decimal String(number=w1699) -> (decimal integer string=w1702:string)  [unwired: 1 in]
              n374 = call "Build_ERD_Header_String_Array.vi"("ERD Name Array In"=w1710, "ERD Number Array In"=w1709, "ERD Name List"=string[] ["Ramp Time"], "New Header?"=w1706, "ERD Number"=w1705) -> ("ERD Name Array Out"=w1708:string[], "ERD Number Array Out"=w1707:string[])  [unwired: 13 in]
              n375 = Insert Into Array(array=w1701, new element=w1702) -> (w1700:string[])  [unwired: 1 in]
            }
            frame 61602 {
              n376 = Decimal String To Number(string=w1739) -> (number=w1740:i32)  [unwired: 2 in, 1 out]
              n377 = To Unsigned Word Integer(number=w1740) -> (unsigned 16bit integer=w1723:u16)
              n378 = Bundle By Name(cluster=w1728, "Coast Time"=w1723) -> (w1727:T7)
              n379 = Number To Decimal String(number=w1723) -> (decimal integer string=w1726:string)  [unwired: 1 in]
              n380 = call "Build_ERD_Header_String_Array.vi"("ERD Name Array In"=w1734, "ERD Number Array In"=w1733, "ERD Name List"=string[] ["Coast Time"], "New Header?"=w1730, "ERD Number"=w1729) -> ("ERD Name Array Out"=w1732:string[], "ERD Number Array Out"=w1731:string[])  [unwired: 13 in]
              n381 = Insert Into Array(array=w1725, new element=w1726) -> (w1724:string[])  [unwired: 1 in]
            }
            frame 61603 {
              n382 = Decimal String To Number(string=w1767) -> (number=w1770:i32)  [unwired: 2 in, 1 out]
              n383 = To Double Precision Float(number=w1770) -> (double precision float=w1769:dbl)
              n384 = Divide(x=w1769, y=32.0) -> (x/y=w1747:dbl)
              n385 = Bundle By Name(cluster=w1759, "Dry Load Size"=w1747) -> (w1758:T7)
              n386 = call "Build_ERD_Header_String_Array.vi"("ERD Name Array In"=w1753, "ERD Number Array In"=w1752, "ERD Name List"=string[] ["Dry Load Size"], "New Header?"=w1749, "ERD Number"=w1748) -> ("ERD Name Array Out"=w1751:string[], "ERD Number Array Out"=w1750:string[])  [unwired: 13 in]
              n387 = Number To Fractional String(number=w1747) -> (F-format string=w1757:string)  [unwired: 3 in]
              n388 = Insert Into Array(array=w1756, new element=w1757) -> (w1755:string[])  [unwired: 1 in]
              n389 = Bundle By Name(cluster=w1766, "Dry Load Size"=w1747) -> (w1765:T3)
            }
            frame 61605 {
              n390 = String Subset(string=w1790, offset (0)=0, length (rest)=2 ("length (rest)")) -> (substring=w1800:string)
              n391 = String Subset(string=w1790, offset (0)=3, length (rest)=2 ("length (rest)")) -> (substring=w1799:string)
              n392 = String Subset(string=w1790, offset (0)=6, length (rest)=2 ("length (rest)")) -> (substring=w1792:string)
              n393 = String Subset(string=w1790, offset (0)=9, length (rest)=2 ("length (rest)")) -> (substring=w1791:string)
              n394 = Concatenate Strings(w1800, w1799, w1792, w1791) -> (w1798:string)
              n395 = Hexadecimal String To Number(string=w1798) -> (number=w1797:u32)  [unwired: 2 in, 1 out]
              n396 = To Long Integer(number=w1797) -> (32bit integer=w1774:i32)
              n397 = call "Build_ERD_Header_String_Array.vi"("ERD Name Array In"=w1785, "ERD Number Array In"=w1784, "ERD Name List"=string[] ["Max Jerk in Accel"], "New Header?"=w1781, "ERD Number"=w1780) -> ("ERD Name Array Out"=w1783:string[], "ERD Number Array Out"=w1782:string[])  [unwired: 13 in]
              n398 = Bundle By Name(cluster=w1806, "Max Jerk in Accel"=w1774) -> (w1805:T4)
              n399 = Number To Decimal String(number=w1774) -> (decimal integer string=w1777:string)  [unwired: 1 in]
              n400 = Insert Into Array(array=w1776, new element=w1777) -> (w1775:string[])  [unwired: 1 in]
              n401 = Bundle By Name(cluster=w1779, "Max Jerk in Accel"=w1774) -> (w1778:T7)
            }
            frame 61606 {
              n402 = String Subset(string=w1828, offset (0)=0, length (rest)=2 ("length (rest)")) -> (substring=w1838:string)
              n403 = String Subset(string=w1828, offset (0)=3, length (rest)=2 ("length (rest)")) -> (substring=w1837:string)
              n404 = String Subset(string=w1828, offset (0)=6, length (rest)=2 ("length (rest)")) -> (substring=w1830:string)
              n405 = String Subset(string=w1828, offset (0)=9, length (rest)=2 ("length (rest)")) -> (substring=w1829:string)
              n406 = Concatenate Strings(w1838, w1837, w1830, w1829) -> (w1836:string)
              n407 = Hexadecimal String To Number(string=w1836) -> (number=w1835:u32)  [unwired: 2 in, 1 out]
              n408 = To Long Integer(number=w1835) -> (32bit integer=w1812:i32)
              n409 = call "Build_ERD_Header_String_Array.vi"("ERD Name Array In"=w1823, "ERD Number Array In"=w1822, "ERD Name List"=string[] ["Max Jerk in S-S"], "New Header?"=w1819, "ERD Number"=w1818) -> ("ERD Name Array Out"=w1821:string[], "ERD Number Array Out"=w1820:string[])  [unwired: 13 in]
              n410 = Bundle By Name(cluster=w1844, "Max Jerk in S-S"=w1812) -> (w1843:T4)
              n411 = Number To Decimal String(number=w1812) -> (decimal integer string=w1817:string)  [unwired: 1 in]
              n412 = Insert Into Array(array=w1816, new element=w1817) -> (w1815:string[])  [unwired: 1 in]
              n413 = Bundle By Name(cluster=w1814, "Max Jerk in S-S"=w1812) -> (w1813:T7)
            }
            frame 61608 {
              n414 = call <vilib>:"Space Constant.vi"() -> ("String"=w1852:string)
              n415 = Search and Replace String(replace all?=TRUE ("replace all? (F)"), input string=w1847, search string=w1852, replace string="" ("replace string (\"\")")) -> (result string=w1850:string)  [unwired: 4 in, 3 out]
              n416 = Hexadecimal String To Number(string=w1850) -> (number=w1848:u32)  [unwired: 2 in, 1 out]
              n417 = Bundle By Name(cluster=w1870, "Shaft Speed"=w1848) -> (w1869:T4)
              n418 = Number To Decimal String(number=w1848) -> (decimal integer string=w1856:string)  [unwired: 1 in]
              n419 = call "Build_ERD_Header_String_Array.vi"("ERD Name Array In"=w1867, "ERD Number Array In"=w1866, "ERD Name List"=string[] ["Shaft Speed"], "New Header?"=w1863, "ERD Number"=w1862) -> ("ERD Name Array Out"=w1865:string[], "ERD Number Array Out"=w1864:string[])  [unwired: 13 in]
              n420 = Insert Into Array(array=w1858, new element=w1856) -> (w1857:string[])  [unwired: 1 in]
              n421 = Bundle By Name(cluster=w1874, "Shaft Speed (RPM)"=w1848) -> (w1873:T3)
            }
            frame 8236 {
              n422 = call "String Remove All Spaces.vi"("Input String"=w1875) -> ("Spaces Removed"=w1876:string)  [unwired: 13 in, 1 out]
              n423 = Hexadecimal String To Number(string=w1876) -> (number=w1900:u32)  [unwired: 2 in, 1 out]
              n424 = To Unsigned Word Integer(number=w1900) -> (unsigned 16bit integer=w1886:u16)
              n425 = Number To Decimal String(number=w1886) -> (decimal integer string=w1880:string)  [unwired: 1 in]
              n426 = call "Build_ERD_Header_String_Array.vi"("ERD Name Array In"=w1892, "ERD Number Array In"=w1891, "ERD Name List"=string[] ["Basket Speed"], "New Header?"=w1888, "ERD Number"=w1887) -> ("ERD Name Array Out"=w1890:string[], "ERD Number Array Out"=w1889:string[])  [unwired: 13 in]
              n427 = Insert Into Array(array=w1882, new element=w1880) -> (w1881:string[])  [unwired: 1 in]
              n428 = Bundle By Name(cluster=w1895, "Basket Speed"=w1886) -> (w1894:T4)
              n429 = Bundle By Name(cluster=w1899, "Basket Speed (RPM)"=w1886) -> (w1897:T3)
            }
            frame 61611 {
              n430 = Decimal String To Number(string=w1922) -> (number=w1923:i32)  [unwired: 2 in, 1 out]
              n431 = To Double Precision Float(number=w1923) -> (double precision float=w1924:dbl)
              n432 = Divide(x=w1924, y=1024.0) -> (x/y=w1904:dbl)
              n433 = call "Build_ERD_Header_String_Array.vi"("ERD Name Array In"=w1913, "ERD Number Array In"=w1912, "ERD Name List"=string[] ["Current RMS (A)"], "New Header?"=w1909, "ERD Number"=w1908) -> ("ERD Name Array Out"=w1911:string[], "ERD Number Array Out"=w1910:string[])  [unwired: 13 in]
              n434 = Number To Fractional String(number=w1904) -> (F-format string=w1907:string)  [unwired: 3 in]
              n435 = Insert Into Array(array=w1906, new element=w1907) -> (w1905:string[])  [unwired: 1 in]
              n436 = Bundle By Name(cluster=w1926, "Current RMS (Amps)"=w1904) -> (w1925:T3)
            }
            frame 8235 {
              n437 = String Subset(string=w1950, offset (0)=0, length (rest)=2 ("length (rest)")) -> (substring=w1956:string)
              n438 = String Subset(string=w1950, offset (0)=3, length (rest)=2 ("length (rest)")) -> (substring=w1955:string)
              n439 = Concatenate Strings(w1956, w1955) -> (w1954:string)
              n440 = Hexadecimal String To Number(string=w1954) -> (number=w1953:u32)  [unwired: 2 in, 1 out]
              n441 = To Word Integer(number=w1953) -> (16bit integer=w1952:i16)
              n442 = Absolute Value(x=w1952) -> (abs(x)=w1951:i16)
              n443 = To Unsigned Word Integer(number=w1951) -> (unsigned 16bit integer=w1936:u16)
              n444 = call "Build_ERD_Header_String_Array.vi"("ERD Name Array In"=w1942, "ERD Number Array In"=w1941, "ERD Name List"=string[] ["Target Speed"], "New Header?"=w1938, "ERD Number"=w1937) -> ("ERD Name Array Out"=w1940:string[], "ERD Number Array Out"=w1939:string[])  [unwired: 13 in]
              n445 = Bundle By Name(cluster=w1945, "Target Speed"=w1936) -> (w1944:T4)
              n446 = Number To Decimal String(number=w1936) -> (decimal integer string=w1931:string)  [unwired: 1 in]
              n447 = Insert Into Array(array=w1932, new element=w1931) -> (w1930:string[])  [unwired: 1 in]
              n448 = Bundle By Name(cluster=w1948, "Target Speed (RPM)"=w1936) -> (w1947:T3)
            }
            frame 61617 {
              n449 = Decimal String To Number(string=w1980) -> (number=w1981:i32)  [unwired: 2 in, 1 out]
              n450 = case shown="0, Default" w1981 {
                tunnel: ["Closed Loop" "Closed Loop Angle" "Open Loop" "Open Loop Angle" "Coasting" "Braking" "Idle"] -> w1971
                frame 0, Default {
                }
                frame 1 {
                }
                frame 2 {
                }
                frame 3 {
                }
                frame 4 {
                }
                frame 5 {
                }
                frame 6 {
                }
              }
              n451 = call "Build_ERD_Header_String_Array.vi"("ERD Name Array In"=w1969, "ERD Number Array In"=w1968, "ERD Name List"=string[] ["Motor Mode"], "New Header?"=w1965, "ERD Number"=w1964) -> ("ERD Name Array Out"=w1967:string[], "ERD Number Array Out"=w1966:string[])  [unwired: 13 in]
              n452 = Insert Into Array(array=w1973, new element=w1971) -> (w1972:string[])  [unwired: 1 in]
              n453 = Bundle By Name(cluster=w1983, "Motor Mode"=w1971) -> (w1982:T3)
            }
            frame 61619 {
              n454 = call "HexStringToBoolean.vi"("Hex String"=w2015) -> ("Boolean"=w1994:bool)
              n455 = Bundle By Name(cluster=w2012, "OOB Detected in Accel"=w1994) -> (w2011:T4)
              n456 = Boolean To (0,1)(Boolean=w1994) -> (0, 1=w1999:i16)
              n457 = call "Build_ERD_Header_String_Array.vi"("ERD Name Array In"=w2006, "ERD Number Array In"=w2005, "ERD Name List"=string[] ["OOB Detected in Accel"], "New Header?"=w2002, "ERD Number"=w2001) -> ("ERD Name Array Out"=w2004:string[], "ERD Number Array Out"=w2003:string[])  [unwired: 13 in]
              n458 = Number To Decimal String(number=w1999) -> (decimal integer string=w2000:string)  [unwired: 1 in]
              n459 = Insert Into Array(array=w1998, new element=w2000) -> (w1997:string[])  [unwired: 1 in]
              n460 = Bundle By Name(cluster=w1996, "OOB Detected in Accel"=w1994) -> (w1995:T7)
            }
            frame 61620 {
              n461 = call "HexStringToBoolean.vi"("Hex String"=w2040) -> ("Boolean"=w2019:bool)
              n462 = Bundle By Name(cluster=w2037, "OOB Detected in S-S"=w2019) -> (w2036:T4)
              n463 = Boolean To (0,1)(Boolean=w2019) -> (0, 1=w2024:i16)
              n464 = call "Build_ERD_Header_String_Array.vi"("ERD Name Array In"=w2031, "ERD Number Array In"=w2030, "ERD Name List"=string[] ["OOB Detected in S-S"], "New Header?"=w2027, "ERD Number"=w2026) -> ("ERD Name Array Out"=w2029:string[], "ERD Number Array Out"=w2028:string[])  [unwired: 13 in]
              n465 = Number To Decimal String(number=w2024) -> (decimal integer string=w2025:string)  [unwired: 1 in]
              n466 = Insert Into Array(array=w2023, new element=w2025) -> (w2022:string[])  [unwired: 1 in]
              n467 = Bundle By Name(cluster=w2021, "OOB Detected in S-S"=w2019) -> (w2020:T7)
            }
            frame 61621 {
              n468 = call "HexStringToBoolean.vi"("Hex String"=w2065) -> ("Boolean"=w2044:bool)
              n469 = Bundle By Name(cluster=w2062, "OOB Redist Req"=w2044) -> (w2061:T4)
              n470 = Boolean To (0,1)(Boolean=w2044) -> (0, 1=w2049:i16)
              n471 = call "Build_ERD_Header_String_Array.vi"("ERD Name Array In"=w2056, "ERD Number Array In"=w2055, "ERD Name List"=string[] ["OOB Redist req"], "New Header?"=w2052, "ERD Number"=w2051) -> ("ERD Name Array Out"=w2054:string[], "ERD Number Array Out"=w2053:string[])  [unwired: 13 in]
              n472 = Number To Decimal String(number=w2049) -> (decimal integer string=w2050:string)  [unwired: 1 in]
              n473 = Insert Into Array(array=w2048, new element=w2050) -> (w2047:string[])  [unwired: 1 in]
              n474 = Bundle By Name(cluster=w2046, "OOB Detected in S-S"=w2044) -> (w2045:T7)
            }
            frame 61623 {
              n475 = String Subset(string=w2088, offset (0)=3, length (rest)=2 ("length (rest)")) -> (substring=w2093:string)
              n476 = String Subset(string=w2088, offset (0)=0, length (rest)=2 ("length (rest)")) -> (substring=w2090:string)
              n477 = Hexadecimal String To Number(string=w2090) -> (number=w2089:u32)  [unwired: 2 in, 1 out]
              n478 = case shown="\"0B\"" w2093 {
                tunnel: ["Unknown" ("Profile Status") "Started" ("Profile Status") "Stopped" ("Profile Status") "Paused" ("Profile Status") "Resumed" ("Profile Status") "Selected" ("Profile Status") "Completed" ("Profile Status")] -> w2069
                frame "00", Default {
                }
                frame "06" {
                }
                frame "07" {
                }
                frame "08" {
                }
                frame "09" {
                }
                frame "0A" {
                }
                frame "0B" {
                }
              }
              n479 = Number To Decimal String(number=w2089) -> (decimal integer string=w2070:string)  [unwired: 1 in]
              n480 = call "Build_ERD_Header_String_Array.vi"("ERD Name Array In"=w2079, "ERD Number Array In"=w2078, "ERD Name List"=string[] ["Motor Profile ", "Motor Profile Status"], "New Header?"=w2075, "ERD Number"=w2074) -> ("ERD Name Array Out"=w2077:string[], "ERD Number Array Out"=w2076:string[])  [unwired: 13 in]
              n481 = Insert Into Array(array=w2073, new element=w2070) -> (w2072:string[])  [unwired: 1 in]
              n482 = Bundle By Name(cluster=w2085, "Motor Profile"=w2070, "Motor Profile Status"=w2069) -> (w2084:T4)
              n483 = Insert Into Array(array=w2072, new element=w2069) -> (w2071:string[])  [unwired: 1 in]
              n484 = Bundle By Name(cluster=w2096, "Motor Profile"=w2070, "Motor Profile Status"=w2069) -> (w2097:T3)
            }
            frame 61628 {
              n485 = call "Parse Brass Matrix ERD.vi"("string"=w2128) -> ("Folding"=w2121:i32, "Jerk"=w2120:i32, "Jerk Delta"=w2109:i32)  [unwired: 16 in]
              n486 = call "Build_ERD_Header_String_Array.vi"("ERD Name Array In"=w2122, "ERD Number Array In"=w2126, "ERD Name List"=string[] ["Acceleration", "Jerk", "Jerk Delta"], "New Header?"=w2124, "ERD Number"=w2125) -> ("ERD Name Array Out"=w2119:string[], "ERD Number Array Out"=w2123:string[])  [unwired: 13 in]
              n487 = Number To Decimal String(number=w2121) -> (decimal integer string=w2112:string)  [unwired: 1 in]
              n488 = Number To Decimal String(number=w2120) -> (decimal integer string=w2111:string)  [unwired: 1 in]
              n489 = Number To Decimal String(number=w2109) -> (decimal integer string=w2108:string)  [unwired: 1 in]
              n490 = Bundle By Name(cluster=w2127, "Folding"=w2121, "Jerk"=w2120, "Jerk Delta"=w2109) -> (w2110:T4)
              n491 = Insert Into Array(array=w2114, new element #1=w2112, new element #2=w2111, new element #3=w2108) -> (w2113:string[])  [unwired: 1 in]
            }
            frame 61630 {
              n492 = call "HexStringToBoolean.vi"("Hex String"=w2152) -> ("Boolean"=w2135:bool)
              n493 = call "Build_ERD_Header_String_Array.vi"("ERD Name Array In"=w2144, "ERD Number Array In"=w2143, "ERD Name List"=string[] ["ME Relay"], "New Header?"=w2140, "ERD Number"=w2139) -> ("ERD Name Array Out"=w2142:string[], "ERD Number Array Out"=w2141:string[])  [unwired: 13 in]
              n494 = case shown="True" w2135 {
                tunnel: ["OFF" "ON"] -> w2138
                frame False {
                }
                frame True {
                }
              }
              n495 = Insert Into Array(array=w2137, new element=w2138) -> (w2136:string[])  [unwired: 1 in]
              n496 = Bundle By Name(cluster=w2154, "ME Relay"=w2135) -> (w2153:T3)
            }
            frame 61631 {
              n497 = call "HexStringToBoolean.vi"("Hex String"=w2179) -> ("Boolean"=w2162:bool)
              n498 = call "Build_ERD_Header_String_Array.vi"("ERD Name Array In"=w2169, "ERD Number Array In"=w2168, "ERD Name List"=string[] ["Mode Shift FB"], "New Header?"=w2165, "ERD Number"=w2164) -> ("ERD Name Array Out"=w2167:string[], "ERD Number Array Out"=w2166:string[])  [unwired: 13 in]
              n499 = case shown="False" w2162 {
                tunnel: ["LOW" "HIGH"] -> w2163
                frame False {
                }
                frame True {
                }
              }
              n500 = Insert Into Array(array=w2161, new element=w2163) -> (w2160:string[])  [unwired: 1 in]
              n501 = Bundle By Name(cluster=w2178, "Mode Shift FB"=w2162) -> (w2177:T3)
            }
            frame 61632 {
              n502 = call "HexStringToBoolean.vi"("Hex String"=w2204) -> ("Boolean"=w2192:bool)
              n503 = Bundle By Name(cluster=w2203, "MS Motor"=w2192) -> (w2202:T3)
              n504 = case shown="True" w2192 {
                tunnel: ["OFF" "ON"] -> w2195
                frame False {
                }
                frame True {
                }
              }
              n505 = call "Build_ERD_Header_String_Array.vi"("ERD Name Array In"=w2190, "ERD Number Array In"=w2189, "ERD Name List"=string[] ["Mode Shift Motor"], "New Header?"=w2186, "ERD Number"=w2185) -> ("ERD Name Array Out"=w2188:string[], "ERD Number Array Out"=w2187:string[])  [unwired: 13 in]
              n506 = Insert Into Array(array=w2194, new element=w2195) -> (w2193:string[])  [unwired: 1 in]
            }
            frame 61636 {
              n507 = Decimal String To Number(string=w2229) -> (number=w2232:i32)  [unwired: 2 in, 1 out]
              n508 = To Double Precision Float(number=w2232) -> (double precision float=w2231:dbl)
              n509 = Divide(x=w2231, y=32.0) -> (x/y=w2211:dbl)
              n510 = call "Build_ERD_Header_String_Array.vi"("ERD Name Array In"=w2219, "ERD Number Array In"=w2218, "ERD Name List"=string[] ["Line Voltage"], "New Header?"=w2215, "ERD Number"=w2214) -> ("ERD Name Array Out"=w2217:string[], "ERD Number Array Out"=w2216:string[])  [unwired: 13 in]
              n511 = Number To Fractional String(number=w2211) -> (F-format string=w2223:string)  [unwired: 3 in]
              n512 = Insert Into Array(array=w2222, new element=w2223) -> (w2221:string[])  [unwired: 1 in]
              n513 = Bundle By Name(cluster=w2228, "Line Voltage"=w2211) -> (w2227:T3)
            }
            frame 61638 {
              n514 = Decimal String To Number(string=w2252) -> (number=w2253:i32)  [unwired: 2 in, 1 out]
              n515 = To Unsigned Word Integer(number=w2253) -> (unsigned 16bit integer=w2236:u16)
              n516 = Number To Decimal String(number=w2236) -> (decimal integer string=w2239:string)  [unwired: 1 in]
              n517 = Bundle By Name(cluster=w2241, "Partial Coast Time"=w2236) -> (w2240:T7)
              n518 = Insert Into Array(array=w2238, new element=w2239) -> (w2237:string[])  [unwired: 1 in]
              n519 = call "Build_ERD_Header_String_Array.vi"("ERD Name Array In"=w2247, "ERD Number Array In"=w2246, "ERD Name List"=string[] ["Partial Coast Time"], "New Header?"=w2243, "ERD Number"=w2242) -> ("ERD Name Array Out"=w2245:string[], "ERD Number Array Out"=w2244:string[])  [unwired: 13 in]
            }
            frame 61639 {
              n520 = Decimal String To Number(string=w2277) -> (number=w2278:i32)  [unwired: 2 in, 1 out]
              n521 = To Double Precision Float(number=w2278) -> (double precision float=w2279:dbl)
              n522 = Divide(x=w2279, y=32.0) -> (x/y=w2262:dbl)
              n523 = call "Build_ERD_Header_String_Array.vi"("ERD Name Array In"=w2272, "ERD Number Array In"=w2271, "ERD Name List"=string[] ["Ramp Line Voltage"], "New Header?"=w2261, "ERD Number"=w2260) -> ("ERD Name Array Out"=w2270:string[], "ERD Number Array Out"=w2269:string[])  [unwired: 13 in]
              n524 = Bundle By Name(cluster=w2267, "Ramp Line Voltage"=w2262) -> (w2266:T7)
              n525 = Number To Fractional String(number=w2262) -> (F-format string=w2265:string)  [unwired: 3 in]
              n526 = Insert Into Array(array=w2264, new element=w2265) -> (w2263:string[])  [unwired: 1 in]
            }
            frame 61640 {
              n527 = String Subset(string=w2286, offset (0)=0, length (rest)=2 ("length (rest)")) -> (substring=w2298:string)
              n528 = String Subset(string=w2286, offset (0)=3, length (rest)=2 ("length (rest)")) -> (substring=w2297:string)
              n529 = String Subset(string=w2286, offset (0)=6, length (rest)=2 ("length (rest)")) -> (substring=w2292:string)
              n530 = String Subset(string=w2286, offset (0)=9, length (rest)=2 ("length (rest)")) -> (substring=w2291:string)
              n531 = Concatenate Strings(w2298, w2297, w2292, w2291) -> (w2290:string)
              n532 = Hexadecimal String To Number(string=w2290) -> (number=w2289:u32)  [unwired: 2 in, 1 out]
              n533 = To Long Integer(number=w2289) -> (32bit integer=w2288:i32)
              n534 = Bundle By Name(cluster=w2306, "Folding in Accel"=w2288) -> (w2305:T4)
              n535 = call "Build_ERD_Header_String_Array.vi"("ERD Name Array In"=w2313, "ERD Number Array In"=w2312, "ERD Name List"=string[] ["Folding in Accel"], "New Header?"=w2309, "ERD Number"=w2307) -> ("ERD Name Array Out"=w2311:string[], "ERD Number Array Out"=w2310:string[])  [unwired: 13 in]
              n536 = Number To Decimal String(number=w2288) -> (decimal integer string=w2304:string)  [unwired: 1 in]
              n537 = Insert Into Array(array=w2303, new element=w2304) -> (w2302:string[])  [unwired: 1 in]
            }
            frame 61641 {
              n538 = call "HexStringToBoolean.vi"("Hex String"=w2344) -> ("Boolean"=w2323:bool)
              n539 = Bundle By Name(cluster=w2341, "Suds Abatement Req"=w2323) -> (w2340:T4)
              n540 = Boolean To (0,1)(Boolean=w2323) -> (0, 1=w2328:i16)
              n541 = call "Build_ERD_Header_String_Array.vi"("ERD Name Array In"=w2335, "ERD Number Array In"=w2334, "ERD Name List"=string[] ["Suds Abtmt Req"], "New Header?"=w2331, "ERD Number"=w2330) -> ("ERD Name Array Out"=w2333:string[], "ERD Number Array Out"=w2332:string[])  [unwired: 13 in]
              n542 = Number To Decimal String(number=w2328) -> (decimal integer string=w2329:string)  [unwired: 1 in]
              n543 = Insert Into Array(array=w2327, new element=w2329) -> (w2326:string[])  [unwired: 1 in]
              n544 = Bundle By Name(cluster=w2325, "Suds Abatement Req"=w2323) -> (w2324:T7)
            }
            frame 61645 {
              n545 = call "Parse Accelerometer ERD.vi"("string"=w2368) -> ("Peak Magnitude"=w2360:dbl, "Peak Signal"=w2359:u8, "Peak Direction"=w2350:bool, "Peak Vector"=w2348:dbl)  [unwired: 15 in]
              n546 = case shown="False" w2350 {
                tunnel: ["Negative" "Positive"] -> w2351
                frame False {
                }
                frame True {
                }
              }
              n547 = call "Build_ERD_Header_String_Array.vi"("ERD Name Array In"=w2366, "ERD Number Array In"=w2365, "ERD Name List"=string[] ["Peak Magnitude", "Peak Signal", "Peak Direction", "Peak Vector"], "New Header?"=w2362, "ERD Number"=w2361) -> ("ERD Name Array Out"=w2364:string[], "ERD Number Array Out"=w2363:string[])  [unwired: 13 in]
              n548 = Bundle By Name(cluster=w2370, "Peak Magnitude"=w2360, "Peak Signal"=w2359, "Peak Dir"=w2350, "Peak Vector"=w2348) -> (w2369:T4)
              n549 = Number To Fractional String(number=w2360) -> (F-format string=w2353:string)  [unwired: 3 in]
              n550 = Number To Decimal String(number=w2359) -> (decimal integer string=w2352:string)  [unwired: 1 in]
              n551 = Number To Fractional String(number=w2348) -> (F-format string=w2349:string)  [unwired: 3 in]
              n552 = Insert Into Array(array=w2355, new element #1=w2353, new element #2=w2352, new element #3=w2351, new element #4=w2349) -> (w2354:string[])  [unwired: 1 in]
            }
            frame 61697 {
              n553 = Decimal String To Number(string=w2379) -> (number=w2396:i32)  [unwired: 2 in, 1 out]
              n554 = To Unsigned Byte Integer(number=w2396) -> (unsigned 8bit integer=w2380:u8)
              n555 = Bundle By Name(cluster=w2382, "Points"=w2380) -> (w2381:T4)
              n556 = call "Build_ERD_Header_String_Array.vi"("ERD Name Array In"=w2388, "ERD Number Array In"=w2387, "ERD Name List"=string[] ["Accelerometer Points"], "New Header?"=w2384, "ERD Number"=w2383) -> ("ERD Name Array Out"=w2386:string[], "ERD Number Array Out"=w2385:string[])  [unwired: 13 in]
              n557 = Insert Into Array(array=w2391, new element=w2379) -> (w2390:string[])  [unwired: 1 in]
            }
            frame 61698 {
              n558 = Decimal String To Number(string=w2402) -> (number=w2419:i32)  [unwired: 2 in, 1 out]
              n559 = To Unsigned Byte Integer(number=w2419) -> (unsigned 8bit integer=w2403:u8)
              n560 = Bundle By Name(cluster=w2405, "S-S Points"=w2403) -> (w2404:T4)
              n561 = call "Build_ERD_Header_String_Array.vi"("ERD Name Array In"=w2411, "ERD Number Array In"=w2410, "ERD Name List"=string[] ["S-S Points"], "New Header?"=w2407, "ERD Number"=w2406) -> ("ERD Name Array Out"=w2409:string[], "ERD Number Array Out"=w2408:string[])  [unwired: 13 in]
              n562 = Insert Into Array(array=w2414, new element=w2402) -> (w2413:string[])  [unwired: 1 in]
            }
            frame 65280 {
              n563 = Build Array("Personality" ("String")) -> (w2423:string[])
              n564 = Decimal String To Number(string=w2440) -> (number=w2441:i32)  [unwired: 2 in, 1 out]
              n565 = To Unsigned Byte Integer(number=w2441) -> (unsigned 8bit integer=w2427:u8)
              n566 = call "Build_ERD_Header_String_Array.vi"("ERD Name Array In"=w2436, "ERD Number Array In"=w2435, "ERD Name List"=w2423, "New Header?"=w2432, "ERD Number"=w2431) -> ("ERD Name Array Out"=w2434:string[], "ERD Number Array Out"=w2433:string[])  [unwired: 13 in]
              n567 = Number To Decimal String(number=w2427) -> (decimal integer string=w2430:string)  [unwired: 1 in]
              n568 = Insert Into Array(array=w2429, new element=w2430) -> (w2428:string[])  [unwired: 1 in]
            }
            frame 51 {
              # "Line Number"
              # "File Name *Last 20 Characters*"
              n569 = String Subset(string=w2453, offset (0)=0, length (rest)=59 ("length (rest)")) -> (substring=w2451:string)
              n570 = call "String Remove All Spaces.vi"("Input String"=w2451) -> ("Spaces Removed"=w2452:string)  [unwired: 13 in, 1 out]
              n571 = call "HexString to AsciiString.vi"("Hex String"=w2452) -> ("ASCII String"=w2450:string)  [unwired: 13 in, 1 out]
              n572 = String Subset(string=w2453, offset (0)=60, length (rest)=2 ("length (rest)")) -> (substring=w2475:string)
              n573 = String Subset(string=w2453, offset (0)=63, length (rest)=2 ("length (rest)")) -> (substring=w2476:string)
              n574 = call "Build_ERD_Header_String_Array.vi"("ERD Name Array In"=w2462, "ERD Number Array In"=w2461, "ERD Name List"=string[] ["Reset Source"], "New Header?"=w2458, "ERD Number"=w2457) -> ("ERD Name Array Out"=w2460:string[], "ERD Number Array Out"=w2459:string[])  [unwired: 13 in]
              n575 = Concatenate Strings(w2475, w2476) -> (w2477:string)
              n576 = Hexadecimal String To Number(string=w2477) -> (number=w2469:u32)  [unwired: 2 in, 1 out]
              n577 = Number To Decimal String(number=w2469) -> (decimal integer string=w2448:string)  [unwired: 1 in]
              n578 = call <vilib>:"Space Constant.vi"() -> ("String"=w2470:string)
              n579 = Concatenate Strings(w2450, w2470, "Line " ("string"), w2448) -> (w2454:string)
              n580 = Bundle By Name(cluster=w2468, "Reset Source"=w2454) -> (w2467:T3)
              n581 = Insert Into Array(array=w2456, new element=w2454) -> (w2455:string[])  [unwired: 1 in]
            }
            frame 65314 {
              n582 = Decimal String To Number(string=w2502) -> (number=w2503:i32)  [unwired: 2 in, 1 out]
              n583 = case shown="4" w2503 {
                tunnel: ["Unknown" ("Motor Profile") "Agitate State" ("Motor Profile") "Spin State" ("Motor Profile") "Trans to Spin" ("Motor Profile") "Trans to Agitate" ("Motor Profile")] -> w2486
                frame 0, Default {
                }
                frame 1 {
                }
                frame 2 {
                }
                frame 3 {
                }
                frame 4 {
                }
              }
              n584 = call "Build_ERD_Header_String_Array.vi"("ERD Name Array In"=w2494, "ERD Number Array In"=w2493, "ERD Name List"=string[] ["Mode Shift Status"], "New Header?"=w2490, "ERD Number"=w2489) -> ("ERD Name Array Out"=w2492:string[], "ERD Number Array Out"=w2491:string[])  [unwired: 13 in]
              n585 = Insert Into Array(array=w2488, new element=w2486) -> (w2487:string[])  [unwired: 1 in]
              n586 = Bundle By Name(cluster=w2505, "Mode Shift Status"=w2486) -> (w2504:T3)
            }
            frame 57 {
              n587 = call "VersionConversionData.vi"("Version In"=w2512) -> ("Version Out"=w2511:string)  [unwired: 9 in, 1 out]
              n588 = call "Build_ERD_Header_String_Array.vi"("ERD Name Array In"=w2527, "ERD Number Array In"=w2526, "ERD Name List"=string[] ["Bootloader Version "], "New Header?"=w2525, "ERD Number"=u16 57) -> ("ERD Name Array Out"=w2524:string[], "ERD Number Array Out"=w2523:string[])  [unwired: 13 in]
              n589 = Bundle By Name(cluster=w2515, "MC BL Version"=w2511) -> (w2514:T13)
              n590 = Insert Into Array(array=w2522, new element=w2511) -> (w2521:string[])  [unwired: 1 in]
            }
            frame 8398 {
              n591 = case shown="\"00\"" w2536 {
                tunnel: ["01_LOCKED" ("Write Access") "FF_REQUESTED" ("Write Access") "00_UNLOCKED" ("Write Access")] -> w2533
                frame "01" {
                }
                frame "FF", Default {
                }
                frame "00" {
                }
              }
              n592 = call "Build_ERD_Header_String_Array.vi"("ERD Name Array In"=w2548, "ERD Number Array In"=w2547, "ERD Name List"=w2534, "New Header?"=w2546, "ERD Number"=w2545) -> ("ERD Name Array Out"=w2544:string[], "ERD Number Array Out"=w2543:string[])  [unwired: 13 in]
              n593 = Bundle By Name(cluster=w2540, "Write Access Actual"=w2533) -> (w2539:T11)
              n594 = Insert Into Array(array=w2538, new element=w2533) -> (w2537:string[])  [unwired: 1 in]
            }
            frame 8397 {
              n595 = case shown="\"00\"" w2561 {
                tunnel: ["01_LOCKED" ("Write Access") "FF_REQUESTED" ("Write Access") "00_UNLOCKED" ("Write Access")] -> w2558
                frame "01" {
                }
                frame "FF", Default {
                }
                frame "00" {
                }
              }
              n596 = call "Build_ERD_Header_String_Array.vi"("ERD Name Array In"=w2573, "ERD Number Array In"=w2572, "ERD Name List"=w2559, "New Header?"=w2571, "ERD Number"=w2570) -> ("ERD Name Array Out"=w2569:string[], "ERD Number Array Out"=w2568:string[])  [unwired: 13 in]
              n597 = Bundle By Name(cluster=w2565, "Write Access Request"=w2558) -> (w2564:T11)
              n598 = Insert Into Array(array=w2563, new element=w2558) -> (w2562:string[])  [unwired: 1 in]
            }
            frame 65356 {
              n599 = case shown="\"01\"" w2586 {
                tunnel: ["01_LOCKED" ("Write Access") "Unknown" ("Write Access") "00_UNLOCKED" ("Write Access")] -> w2583
                frame "01" {
                }
                frame "FF", Default {
                }
                frame "00" {
                }
              }
              n600 = call "Build_ERD_Header_String_Array.vi"("ERD Name Array In"=w2598, "ERD Number Array In"=w2597, "ERD Name List"=w2584, "New Header?"=w2596, "ERD Number"=w2595) -> ("ERD Name Array Out"=w2594:string[], "ERD Number Array Out"=w2593:string[])  [unwired: 13 in]
              n601 = Bundle By Name(cluster=w2590, "LockedAtLeastOnce"=w2583) -> (w2589:T11)
              n602 = Insert Into Array(array=w2588, new element=w2583) -> (w2587:string[])  [unwired: 1 in]
            }
            frame 8351 {
              n603 = String Subset(string=w2609, offset (0)=21, length (rest)=2 ("length (rest)")) -> (substring=w2614:string)
              n604 = String Subset(string=w2609, offset (0)=12, length (rest)=2 ("length (rest)")) -> (substring=w2626:string)
              n605 = String Subset(string=w2609, offset (0)=18, length (rest)=2 ("length (rest)")) -> (substring=w2618:string)
              n606 = String Subset(string=w2609, offset (0)=0, length (rest)=12 ("length (rest)")) -> (substring=w2629:string)
              n607 = String Subset(string=w2609, offset (0)=15, length (rest)=2 ("length (rest)")) -> (substring=w2622:string)
              n608 = String Subset(string=w2609, offset (0)=84, length (rest)=2 ("length (rest)")) -> (substring=w2611:string)
              n609 = case shown="\"FF\", Default" w2626 {
                selector: w2626 -> [_ _ _ _ _ _ _ _ _ w2697 _]
                tunnel: ["RESERVED" ("Write Access") "CYCLE REQUEST" ("Write Access") "CYCLE STARTED" ("Write Access") "PAUSED" ("Write Access") "SESSION EXPIRED" ("Write Access") "Authorized" ("Write Access") "DENIED" ("Write Access") "FAULT" ("Write Access") "SESSION CANCELLED" ("Write Access") w2695 "IDLE" ("Write Access")] -> w2625
                frame "01" {
                }
                frame "02" {
                }
                frame "03" {
                }
                frame "04" {
                }
                frame "05" {
                }
                frame "06" {
                }
                frame "07" {
                }
                frame "08" {
                }
                frame "09" {
                }
                frame "FF", Default {
                  n610 = Concatenate Strings(w2697, "UNKNOWN" ("Write Access")) -> (w2695:string)
                }
                frame "00" {
                }
              }
              n611 = case shown="\"FF\", Default" w2622 {
                selector: w2622 -> [w2675 _ _ _ _ _ _ _ _ _ _]
                tunnel: [w2673 "WaterHeater" ("Write Access") "ClothesDryer" ("Write Access") "ClothesWasher" ("Write Access") "Refrigerator" ("Write Access") "Microwave" ("Write Access") "Advantium" ("Write Access") "Dishwasher" ("Write Access") "Oven" ("Write Access") "ElectricRange" ("Write Access") "Gas Range" ("Write Access")] -> w2621
                frame "FF", Default {
                  n612 = Concatenate Strings(w2675, "UNKNOWN" ("Write Access")) -> (w2673:string)
                }
                frame "00" {
                }
                frame "01" {
                }
                frame "02" {
                }
                frame "03" {
                }
                frame "04" {
                }
                frame "05" {
                }
                frame "06" {
                }
                frame "07" {
                }
                frame "08" {
                }
                frame "09" {
                }
              }
              n613 = case shown="\"FF\", Default" w2618 {
                selector: w2618 -> [w2659 _ _ _ _ _ _ _ _ _ _ _ _ _]
                tunnel: [w2657 "NotDefined" ("Write Access") "BasketClean" ("Write Access") "DrainSpin" ("Write Access") "QuickRinse" ("Write Access") "BulkyItems" ("Write Access") "Sanitize" ("Write Access") "TowelsSheets" ("Write Access") "WasherSteamRefresh" ("Write Access") "NormalMixedLoad" ("Write Access") "Whites" ("Write Access") "DarkColors" ("Write Access") "Jeans" ("Write Access") "HandWash" ("Write Access")] -> w2617
                frame "FF", Default {
                  n614 = Concatenate Strings(w2659, "UNKNOWN" ("Write Access")) -> (w2657:string)
                }
                frame "00" {
                }
                frame "01" {
                }
                frame "02" {
                }
                frame "03" {
                }
                frame "04" {
                }
                frame "05" {
                }
                frame "06" {
                }
                frame "07" {
                }
                frame "08" {
                }
                frame "09" {
                }
                frame "10" {
                }
                frame "11" {
                }
                frame "12" {
                }
              }
              n615 = case shown="\"FF\", Default" w2614 {
                selector: w2614 -> [w2653 _ _ _]
                tunnel: [w2651 "UnKnown" ("Write Access") "TopLoad" ("Write Access") "FrontLoad" ("Write Access")] -> w2613
                frame "FF", Default {
                  n616 = Concatenate Strings(w2653, "UNKNOWN" ("Write Access")) -> (w2651:string)
                }
                frame "00" {
                }
                frame "01" {
                }
                frame "02" {
                }
              }
              n617 = call "Build_ERD_Header_String_Array.vi"("ERD Name Array In"=w2644, "ERD Number Array In"=w2643, "ERD Name List"=w2608, "New Header?"=w2642, "ERD Number"=w2641) -> ("ERD Name Array Out"=w2640:string[], "ERD Number Array Out"=w2639:string[])  [unwired: 13 in]
              n618 = Bundle By Name(cluster=w2631, "Session"=w2629, "Phase"=w2625, "Appliance Type"=w2621, "Cycle Selected"=w2617, "Platform Type"=w2613, "Retry Signal"=w2611) -> (w2630:T12)
              n619 = Insert Into Array(array=w2637, new element=w2609) -> (w2636:string[])  [unwired: 1 in]
            }
            frame 8350 {
              n620 = String Subset(string=w2700, offset (0)=21, length (rest)=2 ("length (rest)")) -> (substring=w2705:string)
              n621 = String Subset(string=w2700, offset (0)=12, length (rest)=2 ("length (rest)")) -> (substring=w2717:string)
              n622 = String Subset(string=w2700, offset (0)=18, length (rest)=2 ("length (rest)")) -> (substring=w2709:string)
              n623 = String Subset(string=w2700, offset (0)=0, length (rest)=12 ("length (rest)")) -> (substring=w2720:string)
              n624 = String Subset(string=w2700, offset (0)=15, length (rest)=2 ("length (rest)")) -> (substring=w2713:string)
              n625 = String Subset(string=w2700, offset (0)=84, length (rest)=2 ("length (rest)")) -> (substring=w2702:string)
              n626 = case shown="\"FF\", Default" w2717 {
                selector: w2717 -> [_ _ _ _ _ _ _ _ _ w2788 _]
                tunnel: ["RESERVED" ("Write Access") "CYCLE REQUEST" ("Write Access") "CYCLE STARTED" ("Write Access") "PAUSED" ("Write Access") "SESSION EXPIRED" ("Write Access") "Authorized" ("Write Access") "DENIED" ("Write Access") "FAULT" ("Write Access") "SESSION CANCELLED" ("Write Access") w2786 "IDLE" ("Write Access")] -> w2716
                frame "01" {
                }
                frame "02" {
                }
                frame "03" {
                }
                frame "04" {
                }
                frame "05" {
                }
                frame "06" {
                }
                frame "07" {
                }
                frame "08" {
                }
                frame "09" {
                }
                frame "FF", Default {
                  n627 = Concatenate Strings(w2788, "UNKNOWN" ("Write Access")) -> (w2786:string)
                }
                frame "00" {
                }
              }
              n628 = case shown="\"FF\", Default" w2713 {
                selector: w2713 -> [w2766 _ _ _ _ _ _ _ _ _ _]
                tunnel: [w2764 "WaterHeater" ("Write Access") "ClothesDryer" ("Write Access") "ClothesWasher" ("Write Access") "Refrigerator" ("Write Access") "Microwave" ("Write Access") "Advantium" ("Write Access") "Dishwasher" ("Write Access") "Oven" ("Write Access") "ElectricRange" ("Write Access") "Gas Range" ("Write Access")] -> w2712
                frame "FF", Default {
                  n629 = Concatenate Strings(w2766, "UNKNOWN" ("Write Access")) -> (w2764:string)
                }
                frame "00" {
                }
                frame "01" {
                }
                frame "02" {
                }
                frame "03" {
                }
                frame "04" {
                }
                frame "05" {
                }
                frame "06" {
                }
                frame "07" {
                }
                frame "08" {
                }
                frame "09" {
                }
              }
              n630 = case shown="\"FF\", Default" w2709 {
                selector: w2709 -> [w2750 _ _ _ _ _ _ _ _ _ _ _ _ _]
                tunnel: [w2748 "NotDefined" ("Write Access") "BasketClean" ("Write Access") "DrainSpin" ("Write Access") "QuickRinse" ("Write Access") "BulkyItems" ("Write Access") "Sanitize" ("Write Access") "TowelsSheets" ("Write Access") "WasherSteamRefresh" ("Write Access") "NormalMixedLoad" ("Write Access") "Whites" ("Write Access") "DarkColors" ("Write Access") "Jeans" ("Write Access") "HandWash" ("Write Access")] -> w2708
                frame "FF", Default {
                  n631 = Concatenate Strings(w2750, "UNKNOWN" ("Write Access")) -> (w2748:string)
                }
                frame "00" {
                }
                frame "01" {
                }
                frame "02" {
                }
                frame "03" {
                }
                frame "04" {
                }
                frame "05" {
                }
                frame "06" {
                }
                frame "07" {
                }
                frame "08" {
                }
                frame "09" {
                }
                frame "10" {
                }
                frame "11" {
                }
                frame "12" {
                }
              }
              n632 = case shown="\"FF\", Default" w2705 {
                selector: w2705 -> [w2744 _ _ _]
                tunnel: [w2742 "UnKnown" ("Write Access") "TopLoad" ("Write Access") "FrontLoad" ("Write Access")] -> w2704
                frame "FF", Default {
                  n633 = Concatenate Strings(w2744, "UNKNOWN" ("Write Access")) -> (w2742:string)
                }
                frame "00" {
                }
                frame "01" {
                }
                frame "02" {
                }
              }
              n634 = call "Build_ERD_Header_String_Array.vi"("ERD Name Array In"=w2735, "ERD Number Array In"=w2734, "ERD Name List"=w2699, "New Header?"=w2733, "ERD Number"=w2732) -> ("ERD Name Array Out"=w2731:string[], "ERD Number Array Out"=w2730:string[])  [unwired: 13 in]
              n635 = Bundle By Name(cluster=w2722, "Session Ext"=w2720, "Phase Ext"=w2716, "Appliance Type Ext"=w2712, "Cycle Selected Ext"=w2708, "Platform Type Ext"=w2704, "Retry Signal Ext"=w2702) -> (w2721:T12)
              n636 = Insert Into Array(array=w2728, new element=w2700) -> (w2727:string[])  [unwired: 1 in]
            }
          }
        }
        n637 = in-place-cluster #1("CSV File String Arrays.ERD Name Array"=w29, "CSV File String Arrays.ERD Number Array"=w28, "Software MC"=w39, "Brass Matrix"=w38, "ERD_Always Show"=w37, "Personality Set"=w35, "Redundant Micro"=w27, "Algorithm Data"=w24, "ATC Data"=w22, "CSV File String Arrays.ERD Converted String Data"=w30, "RJ45"=w20, "Commercial_Laundry"=w18, "Boot Loader Version"=w16) -> (w10:T1)
      }
    }
    frame Error {
      n638 = Unbundle By Name(w2792) -> ("code"=w2796:i32, "status"=w2797:bool, "source"=w2794:string)
      n639 = Equal?(x=w2796, y=-5006) -> (x = y?=w2800:bool)
      n640 = case shown="True" w2800 {
        tunnel: [w2804 FALSE] -> w2798
        tunnel: w2797 -> [w2804 _]
        tunnel: w2796 -> [w2803 w2806]
        tunnel: [w2803 w2806] -> w2795
        tunnel: [w2802 w2805] -> w2793
        tunnel: w2794 -> [w2802 w2805]
        frame False {
        }
        frame True {
        }
      }
      n641 = Bundle By Name(cluster=errorcluster {"status"=FALSE, "code"=0, "source"=""} ("error constant"), "status"=w2798, "code"=w2795, "source"=w2793) -> (w2791:errorcluster)
    }
  }
  "Error Out" <- w5
  "All_ERD_Data_Bundled_Brass" <- w4
